vi "Versa_06.vi"() -> ()   [LabVIEW 2020]
uses:
  Visualisierungs Elemente/Zahlen-Ausgabefeld.ctl
  Funktionstasten/Funktionstasten.ctl
  Visualisierungs Elemente/Button.ctl
  Visualisierungs Elemente/String - Ausgabefeld.ctl
  IAG-Logo-A2.ctl
  Funktionstasten/Samplepoint Auswahlfeld.ctl
  Status Analysatoren/Status Analysatoren_Anzeige.ctl
  Seiten/FT-IR/FGV FT-IR Aktionen.ctl
  Funktionstasten/Funktionstasten-Aktion.ctl
  Passwortverwaltung/FGV Passwort Aktion.ctl
  Status Analysatoren/Aktion Status Analysatoren.ctl
  Auto Kalibrieren/Aktionen Zeitstempel speichern.ctl
  Seiten/Erweiterte Konfig/Aktion LN2 Extern Befuellung Warnung.ctl
  Seiten/System Einstellungen V2/Aktioen FGV System Konstanten.ctl
  SysLog/Aktionen FGV SysLog.ctl
  Funktionstasten/Zustaende.ctl
  Funktionstasten/Freigabe Aktionen.ctl
  Sprachverwaltung/FGV Aktion Tabelle zerlegen.ctl
  Allgemein/Aktion FGV Aufheizphase.ctl
  Allgemein/AufheizphaseCluster.ctl
  SysLog/SysLog Interface.ctl
  Funktionstasten/Aktionen Zustaende Loggen.ctl
  Stoerungen/Stoerungen Messgeraet/Aktionen Kommunikation Stoerung.ctl
  Allgemein/Aktionen Daten am cRIO speichern.ctl
  Seiten/Erweiterte Konfig/Aktionen LN2 Dewar Spuelen.ctl
  EPA 1065/Allgemeine VIs/Aktion Test Status.ctl
  <vilib>/event_ctls.llb/eventvkey.ctl
  Seiten/Log Konfig/Aktionen Trigger.ctl
  Bildwechsel/Bild-Auswahl.ctl
  Seiten/Anlagengrenzwerte/Aktion Durchflussaenderung.ctl
  Seiten/EL3000/FID/Aktion STY_MES.ctl
  Funktionstasten/FGV Erweiterte Bedienung Aktion.ctl
  AK-Schnittstelle/AK SATK Aktion.ctl
  Seiten/System Einstellungen V2/Aktioen FGV System.ctl
  Allgemein/Zykluszeiterfassung Aktionen.ctl
  Stoerungen/FGV Stoerungsdatei Aktionen.ctl
  Allgemein/Betriebsdaten Aktionen.ctl
  AK-Schnittstelle/AK Namen Aktionen.ctl
  Seiten/FT-IR/FGV FT-IR Gasliste Aktionen.ctl
  Seiten/CalGas Aufschaltung/FGV CalGas Aktionen.ctl
  Seiten/CalGas Aufschaltung/Cluster Auswahl Analysator.ctl
  Seiten/CalGas Aufschaltung/Analysator Auswahl.ctl
  Seiten/FT-IR/TOOLweb Interface Library/Trigger Aktionen.ctl
  Seiten/CalGas Aufschaltung/Definition CalGas Anzeige.ctl
  Seiten/CalGas Aufschaltung/CalGas-Namen.ctl
  Visualisierungs Elemente/String - Eingabefeld.ctl
  Seiten/CalGas Aufschaltung/CalGas-Werte.ctl
  Visualisierungs Elemente/Zahlen-Eingabefeld.ctl
  Seiten/CalGas Aufschaltung/CalGas-Einheit.ctl
  Visualisierungs Elemente/Auswahlfeld.ctl
  Seiten/CalGas Aufschaltung/CalGas-Messbereiche.ctl
  Schedule Modul/Aktion FGV Scheduler Status.ctl
  Stoerungen/FGV Stoermeldungen Aktion.ctl
  Allgemein/Bitte Warten.vi
  Passwortverwaltung/VI Passwortverwaltung.vi
  SysLog/SysLog Status.vi
  Sprachverwaltung/SprachEditor.vi
  Backup mit WebDAV/Backup.vi
  Allgemein/SPRACHE.vi
  EPA 1065/Dichtheitstest 1065-345/Konfig Leak Check.vi
  EPA 1065/Interference verificaton 1065-366/VI Interference Konfig.vi
  EPA 1065/T90 1065-308/T90 Test Konfig.vi
  EPA 1065/Interference verificaton 1065-375/VI Interference Konfig.vi
  EPA 1065/Gas Analyzer Drift 1065-550/Drift Verification Konfig.vi
  Linearisierung V2/VI Linearisierung v2.vi
  EPA 1065/HovaCAL Interference verification/VI Interference Konfig.vi
  Allgemein/allgemeine Sub-VIs.lvlib
  Seiten/FT-IR/TOOLweb Interface Library/TOOLweb Interface.lvlib
  Passwortverwaltung/Passwort.lvlib
  Funktionstasten/Funktionstasten.lvlib
  Bildwechsel/Bildwechsel.lvlib
  cRIO/PC/Kommunikation mit cRIO.lvlib
  Seiten/FT-IR/FT-IR.lvlib
  Seiten/FT-IR/TOOLweb Interface Library/Typdefinitionen.lvlib
  Seiten/Gaszuordnung AO/Gaszuordnung AO.lvlib
  Stoerungen/Stoerungen.lvlib
  Messdaten/Messdaten.lvlib
  AK-Schnittstelle/AK-Schnittstelle.lvlib
  Seiten/Log Konfig/LogKonfig.lvlib
  PNS/Komm Modbus/Komm Modbus.lvlib
  Seiten/Erweiterte Konfig/Erweiterte Konfig.lvlib
  cRIO Ueberwachung/cRIO Ueberwachung.lvlib
  Seiten/System Einstellungen V2/System Einstellungen V2.lvlib
  EPA 1065/Dichtheitstest 1065-345/Dichtheitstest 1065-345.lvlib
  Sprachverwaltung/Sprachverwaltung.lvlib
  Status Analysatoren/Status Analysatoren.lvlib
  Seiten/EL3000/FID/FID.lvlib
  Seiten/EL3000/PMA/PMA.lvlib
  Amium PNS/AK Kommunikation/AK Kommunikation.lvlib
  SysLog/SysLog.lvlib
  Backup mit WebDAV/Backup.lvlib
  Amium PNS/Amium PNS.lvlib
  Amium PNS/Aktion FGV Amium Daten.ctl
  Auto Kalibrieren/VI Auto Kalibrieren.vi
  Auto Kalibrieren/Auto Kalibrieren.lvlib
  Linearisierung V2/Gasteiler/Gasteiler.lvlib
  Linearisierung V2/Gasteiler/HovaCal/HovaCal.lvlib
  FTP WebDAV/FTP WebDAV.lvlib
  Seiten/CalGas Aufschaltung/CalGas Aufschaltung.lvlib
  Seiten/Anlagengrenzwerte/Anlagengrenzwerte.lvlib
  EPA 1065/ANR Test 1065-305/ARN Test 1065-305.lvlib
  EPA 1065/Interference verificaton 1065-366/Interference verificaton 1065-366.lvlib
  EPA 1065/T90 1065-308/T90 Test 1065-308.lvlib
  EPA 1065/EPA 1065.lvlib
  EPA 1065/Interference verificaton 1065-375/Interference verificaton 1065-375.lvlib
  Schedule Modul/Schedule Modul.lvlib
  EPA 1065/Gas Analyzer Drift 1065-550/Gas Analyzer Drift 1065-550.lvlib
  Linearisierung V2/Linearisierung v2.lvlib
  EPA 1065/HovaCAL Interference verification/HovaCAL Interference verificaton.lvlib
panel:
  out "Externe LN2 Warnung":string
  out "TestStatus":string
  in  "Aufschaltung Popup":bool
  in  "SystemLogListe":i32[](listbox)
  in  "SysLog":T1
  in  "Status Analysatoren":T2
  in  "LN2-Behälter Spülen":bool
  out "Letzte Kalibrierung":timestamp format="%<%H:%M:%S\n%x>T"
  out "LifeBit":bool
  in  "Betriebsart":u16(ring) items=["Manuell", "Remote", "Bitparallel"]
  out "Aktuelles Rezept":T3
  out "Datum und Uhrzeit":T3
  in  "login":T1
  out "PW-Level":T4 caption="Password-Level" format="%#_5g"
  in  "Funktionstasten":T5
  in  "Samplepoint":T6 items=["SP1"=1, "SP2"=2]
  in  "IAG":T7
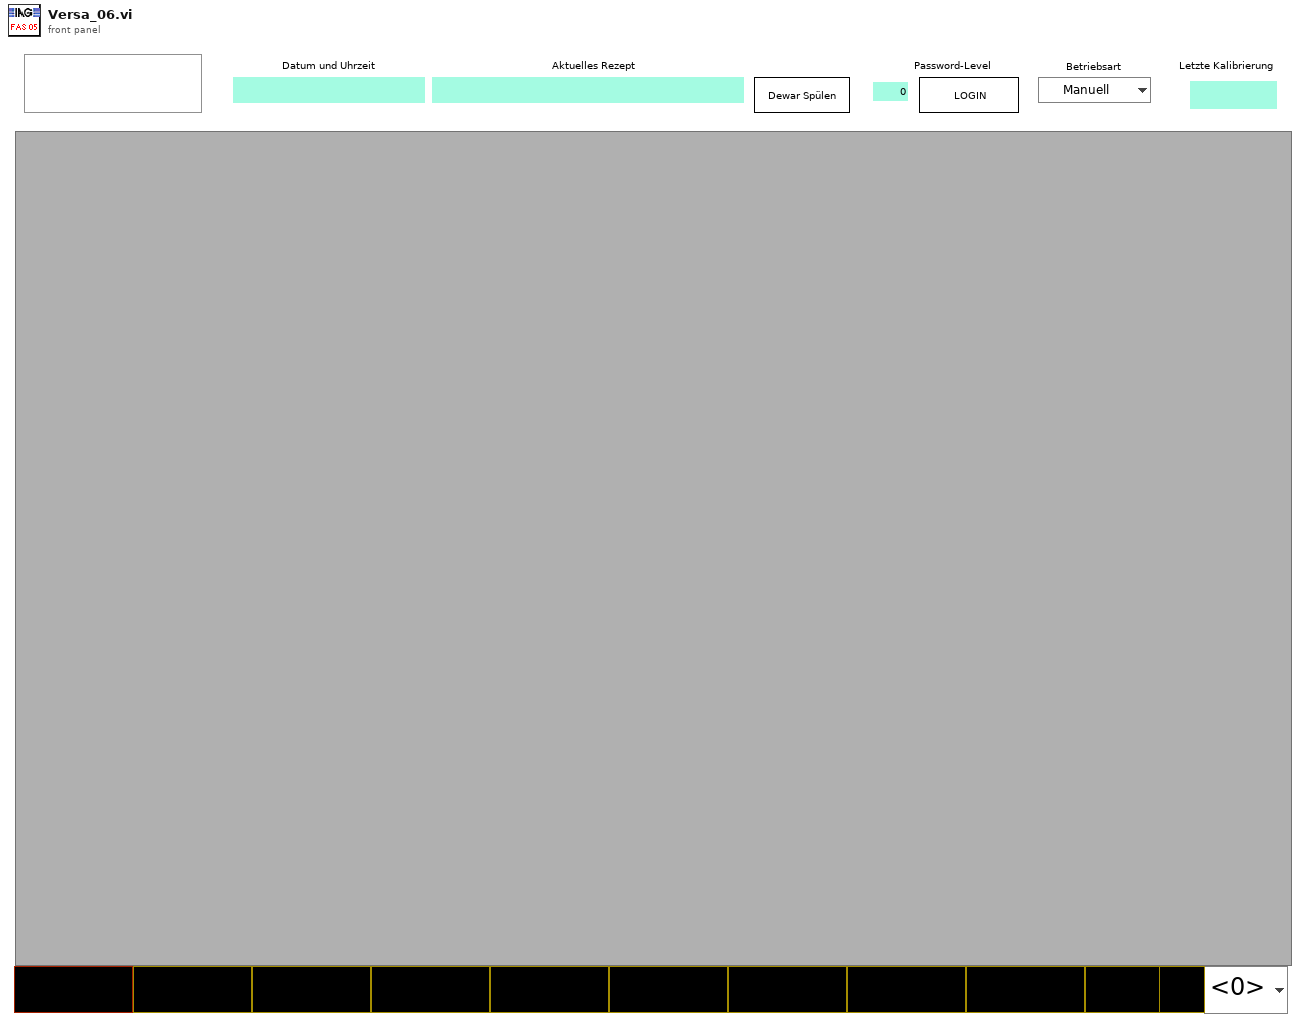
[diagram p1: front panel]
types:
  T1 = typedef "Button.ctl" = bool
  T2 = typedef "Status Analysatoren.lvlib/Status Analysatoren_Anzeige.ctl" = cluster{"FT-IR":bool, "FID":bool, "PMA":bool}
  T3 = typedef "String - Ausgabefeld.ctl" = string
  T4 = typedef "Zahlen-Ausgabefeld.ctl" = sgl
  T5 = typedef "Funktionstasten.lvlib/Funktionstasten.ctl" = cluster{"Taste 1":bool, "Taste 2":bool, "Taste 3":bool, "Taste 4":bool, "Taste 5":bool, "Taste 6":bool, "Taste 7":bool, "Taste 11":bool, "Taste 9":bool, "Taste 10":bool}
  T6 = typedef "Funktionstasten.lvlib/Samplepoint Auswahlfeld.ctl" = u16
  T7 = typedef "IAG-Logo-A2.ctl" = bool
  T8 = typedef "SysLog.lvlib/Aktionen FGV SysLog.ctl" = enum16{"initialisieren", "lesen", "schreiben", "history button ref", "Syslog_Anforderung"}
  T9 = typedef "Erweiterte Konfig.lvlib/Aktion LN2 Extern Befuellung Warnung.ctl" = enum16{"init", "blinken", "Warnungen ausgeben"}
  T10 = typedef "allgemeine Sub-VIs.lvlib/AufheizphaseCluster.ctl" = cluster{"FTIR":bool, "PNS Filterblock":bool, "Versa HL1":bool, "Versa HL2":bool, "PNS HL1":bool, "PNS HL2":bool, "PNS HL3":bool, "PNS HL4":bool, "HL zu FTIR":bool}
  T11 = typedef "allgemeine Sub-VIs.lvlib/Aktion FGV Aufheizphase.ctl" = enum16{"init", "lesen", "PNS Filterblock", "PNS HL1", "PNS HL2", "PNS HL3", "PNS HL4", "FTIR Messzelle", "HL 1", "HL 2", "HL zu FTIR", "auswerten"}
  T12 = typedef "Sprachverwaltung.lvlib/FGV Aktion Tabelle zerlegen.ctl" = enum16{"laden", "vereinzeln", "speichern"}
  T13 = typedef "Status Analysatoren.lvlib/Aktion Status Analysatoren.ctl" = enum16{"lesen", "initialisieren", "Analysatoren aktiv", "FTIR Fehler", "FID Fehler", "PMA Fehler", "Felder einfärben"}
  T14 = typedef "System Einstellungen V2.lvlib/Aktioen FGV System Konstanten.ctl" = enum16{"lesen", "laden", "speichern", "Sprache"}
  T15 = typedef "Funktionstasten.lvlib/Freigabe Aktionen.ctl" = enum16{"prüfen", "Freigabe?", "lesen"}
  T16 = typedef "Funktionstasten.lvlib/Zustaende.ctl" = enum16{"Standby", "Pause", "Eco", "Messen", "Kalibrieren", "Spülen Filter", "Spülen Leitung", "Umgebungsluft", "0-Gas", "Cal-Gas", "CG zu PNS", "-------------", "Init 1", "Init 2", "Init 3", "Init 4", "Messen vorbereiten", "Messen durchführen", "Exit"}
  T17 = typedef "Funktionstasten.lvlib/Funktionstasten-Aktion.ctl" = enum16{"Initialisieren", "Zustand setzen", "Taste gedrückt", "Fehler speichern", "Lesen", "Manuell", "Remote", "Bitparallel", "Samplepoint", "Zeit Prüfen", "reset Umschalten"}
  T18 = typedef "Funktionstasten.lvlib/Aktionen Zustaende Loggen.ctl" = enum16{"lesen", "schreiben", "löschen", "init"}
  T19 = typedef "SysLog.lvlib/SysLog Interface.ctl" = cluster{"FehlermeldungsCode":i32, "ErfolgsmeldungsCode":i32, "ParameterListenString":string, "Anzeige":bool, "SysLogIcon":enum16{"OK", "Warnung", "Fehler"}, "intern":bool}
  T20 = cluster{"Modell":string, "ProjektNummer":string, "Software Version":string, "Seriennummer":string}
  T21 = typedef "allgemeine Sub-VIs.lvlib/Aktionen Daten am cRIO speichern.ctl" = enum16{"lesen", "speichern setzen", "speichern reset", "gespeichert"}
  T22 = cluster{"Anzeige Array":bool[], "Message Array":string[], "SysLog Incon Array":enum16{"OK", "Warnung", "Fehler"}[], "Status Message Array":string[], "Status SysLog Incon Array":enum16{"OK", "Warnung", "Fehler"}[]}
  T23 = typedef "EPA 1065.lvlib/Aktion Test Status.ctl" = enum16{"init", "lesen", "prüfen", "Interference 366", "Interference 375", "Chiller läuft", "Drift läuft", "Pre Test läuft", "FID Optimization läuft", "FID Interference läuft", "HovaCAL Interference", "LinV2"}
  T24 = typedef "Erweiterte Konfig.lvlib/Aktionen LN2 Dewar Spuelen.ctl" = enum16{"lesen", "schreiben", "prüfen"}
  T25 = typedef "System Einstellungen V2.lvlib/Aktioen FGV System.ctl" = enum16{"lesen", "laden", "speichern", "Optionen schreiben", "Zeitstempel", "Reset BMP", "Reset SQP", "Wartung", "Werkseinstellung"}
  T26 = typedef "Amium PNS.lvlib/Aktion FGV Amium Daten.ctl" = enum16{"lesen", "Komm Daten", "Daten", "Error", "Regler", "Grenzwerte", "laden", "speichern"}
  T27 = typedef "eventvkey.ctl" = enum16{"ASCII", "Enter", "Return", "Shift", "Ctrl", "Alt", "Cmd", "Opt", "Caps", "NumLock", "Clear", "Break", "Up", "Down", "Left", "Right", "Insert", "Delete", "Home", "End", "PageUp", "PageDown", "Escape", "Help", "Pause", "ScrollLock", "F1", "F2", "F3", "F4", "F5", "F6", "F7", "F8", "F9", "F10", "F11", "F12", "F13", "F14", "F15", "F16", "F17", "F18", "F19", "F20", "F21", "F22", "F23", "F24", "Play", "VolumeUp", "VolumeDown", "Mute", "Two Byte Char"}
  T28 = typedef "LogKonfig.lvlib/Aktionen Trigger.ctl" = enum16{"lesen", "ALLE schreiben", "Trigger prüfen", "Trigger rücksetzen"}
  T29 = typedef "Bildwechsel.lvlib/Bild-Auswahl.ctl" = enum16{"lesen", "Initialisieren", "Beenden", "Grafik", "Anlagenübersicht", "Anlagengrenzwerte", "Log Konfig", "Gaszuordnung AO", "Erw. Konfiguration", "FT-IR  ", "Störmeldungen", "Störmeldepuffer", "Störmeldekonfig", "PNS Grenzwerte", "Statusübersicht", "Linearisierung", "ARN", "EPA Dichtheitstest", "FID", "PMA", "CalGas", "Lambda", "Interference", "Amium PNS", "EPA T90", "Interference N2O", "Scheduler", "Systemeinstellungen", "EPA Drift", "CAN Konfig", "HovaCAL Interference"}
  T30 = typedef "Passwort.lvlib/FGV Passwort Aktion.ctl" = enum16{"prüfen", "setzen", "Initialisieren", "PW speichern", "lesen", "PW Änderung"}
  T31 = typedef "Anlagengrenzwerte.lvlib/Aktion Durchflussaenderung.ctl" = enum16{"lesen", "Statusänderung", "Reset"}
  T32 = typedef "Aktion STY_MES.ctl" = enum16{"lesen", "setze STY", "setze MES", "MODBUS schreiben"}
  T33 = typedef "AK-Schnittstelle.lvlib/AK SATK Aktion.ctl" = enum16{"initialisieren", "lesen", "schreiben"}
  T34 = typedef "Funktionstasten.lvlib/FGV Erweiterte Bedienung Aktion.ctl" = enum16{"Lesen", "Initialisieren", "N2 zu PNS", "Chart wechsel"}
  T35 = typedef "FT-IR.lvlib/FGV FT-IR Aktionen.ctl" = enum16{"lesen", "NOG setzen", "NOS setzen", "Initialisieren", "speichern", "ALLES setzen", "FT-IR Spektrum loggen", "Komm Stoppen", "Spektrum LogKonfig"}
  T36 = enum16{"startrun", "runonce", "stoprun", "pauserun", "resumerun", "takeback"}
  T37 = typedef "Stoerungen.lvlib/Aktionen Kommunikation Stoerung.ctl" = enum16{"lesen", "init", "FT-IR Komm", "FT-IR Betriebsart", "FT-IR Hintergrund", "cRIO Komm", "PNS Komm", "Dichtheitstest", "Life Bit", "FTIR Komm AK", "PMA Komm", "FID Komm", "PMA Cal", "FID Ch4 Cal", "FID THC Cal", "Cal Timeout", "VFS 1 Komm", "VFS 2 Komm", "VFS 3 Komm", "VFS 4 Komm", "TRE 08 Komm", "CG-Test vorzeitig", "CG-Test Span 1", "CG-Test Span 2", "CG-Test Span 3", "CG-Test Messgas", "CG-Test löschen", "Test", "Amium AK", "AK Recept konfig", "AK Name konfig", "AK EKFG konfig"}
  T38 = enum16{"Init", "scroll H aktiv", "scroll H inaktiv", "scroll V aktiv", "scroll V inaktiv"}
  T39 = typedef "allgemeine Sub-VIs.lvlib/Zykluszeiterfassung Aktionen.ctl" = enum16{"lesen", "init", "Messdaten1", "ToolWeb", "AK FT-IR", "AK Extern", "AK Amium"}
  T40 = typedef "Stoerungen.lvlib/FGV Stoerungsdatei Aktionen.ctl" = enum16{"lesen", "laden", "Neue Werte"}
  T41 = typedef "allgemeine Sub-VIs.lvlib/Betriebsdaten Aktionen.ctl" = enum16{"Laden", "Speichern"}
  T42 = typedef "FT-IR.lvlib/FGV FT-IR Gasliste Aktionen.ctl" = enum16{"lesen", "Gasliste FT-IR", "Gasliste ausgelesen", "laden", "speichern", "löschen"}
  T43 = typedef "AK-Schnittstelle.lvlib/AK Namen Aktionen.ctl" = enum16{"lesen", "laden", "speichern Namen", "AK Namen", "Liste erstellen", "EKFG erstellen", "speichern EKFG", "EKFG schreiben", "Neuen Eintrag erzeugen"}
  T44 = typedef "CalGas Aufschaltung.lvlib/FGV CalGas Aktionen.ctl" = enum16{"lesen", "Analysator Auswahl", "Def.CalGas", "Aufschaltung CalGas", "laden", "speichern", "KAL extrahieren"}
  T45 = typedef "CalGas Aufschaltung.lvlib/Cluster Auswahl Analysator.ctl" = cluster{"Analysator Auswahl":T46, "Analysator Auswahl 2":T46, "Analysator Auswahl 3":T46, "Analysator Auswahl 4":T46, "Analysator Auswahl 5":T46, "Analysator Auswahl 6":T46, "Analysator Auswahl 7":T46, "Analysator Auswahl 8":T46, "Analysator Auswahl 9":T46, "Analysator Auswahl 10":T46, "Analysator Auswahl 11":T46, "Analysator Auswahl 12":T46}
  T46 = typedef "CalGas Aufschaltung.lvlib/Analysator Auswahl.ctl" = u16
  T47 = typedef "Schedule Modul.lvlib/Aktion FGV Scheduler Status.ctl" = enum16{"lesen", "init", "aktiv", "inaktiv"}
  T48 = typedef "CalGas Aufschaltung.lvlib/Definition CalGas Anzeige.ctl" = cluster{"Namen":T49, "Werte":T51, "Werte 2":T51, "Einheit":T53, "Messbereiche":T55}
  T49 = typedef "CalGas Aufschaltung.lvlib/CalGas-Namen.ctl" = cluster{"Name":T50, "Name 2":T50, "Name 3":T50, "Name 4":T50, "Name 5":T50, "Name 6":T50, "Name 7":T50, "Name 8":T50, "Name 9":T50, "Name 10":T50, "Name 11":T50, "Name 12":T50}
  T50 = typedef "String - Eingabefeld.ctl" = string
  T51 = typedef "CalGas Aufschaltung.lvlib/CalGas-Werte.ctl" = cluster{"Konzentration 1":T52, "Konzentration 2":T52, "Konzentration 3":T52, "Konzentration 4":T52, "Konzentration 5":T52, "Konzentration 6":T52, "Konzentration 7":T52, "Konzentration 8":T52, "Konzentration 9":T52, "Konzentration 10":T52, "Konzentration 11":T52, "Konzentration 12":T52}
  T52 = typedef "Zahlen-Eingabefeld.ctl" = sgl
  T53 = typedef "CalGas Aufschaltung.lvlib/CalGas-Einheit.ctl" = cluster{"Einheit 1":T54, "Einheit 2":T54, "Einheit 3":T54, "Einheit 4":T54, "Einheit 5":T54, "Einheit 6":T54, "Einheit 7":T54, "Einheit 8":T54, "Einheit 9":T54, "Einheit 10":T54, "Einheit 11":T54, "Einheit 12":T54}
  T54 = typedef "Auswahlfeld.ctl" = u16
  T55 = typedef "CalGas Aufschaltung.lvlib/CalGas-Messbereiche.ctl" = cluster{"Messbereich 1":T54, "Messbereich 2":T54, "Messbereich 3":T54, "Messbereich 4":T54, "Messbereich 5":T54, "Messbereich 6":T54, "Messbereich 7":T54, "Messbereich 8":T54, "Messbereich 9":T54, "Messbereich 10":T54, "Messbereich 11":T54, "Messbereich 12":T54}
  T56 = typedef "FT-IR.lvlib/TOOLweb Interface.lvlib/Typdefinitionen.lvlib/Trigger Aktionen.ctl" = enum16{"startrun", "runonce", "stoprun", "pauserun", "resumerun", "takeback"}
  T57 = typedef "Stoerungen.lvlib/FGV Stoermeldungen Aktion.ctl" = enum16{"Initialisieren", "kommend", "gehend", "lesen", "Queue leeren", "Queue freigeben", "in Datei loggen", "Änderung zurücksetzen"}
  T58 = typedef "Funktionstasten.lvlib/Betriebsart.ctl" = enum16{"Manuell", "Remote", "Bitparallel"}
  T59 = typedef "Amium PNS.lvlib/Daten Cluster.ctl" = cluster{"Amium Zustände":T60, "Samplepoint am PNS":i16, "Gerätekennung":string, "aktiver Samplepoint":i16[], "Messgasdruck":sgl}
  T60 = typedef "Amium PNS.lvlib/Amium Zustand.ctl" = u16
  T61 = typedef "System Einstellungen V2.lvlib/Optionen.ctl" = cluster{"Störmeldep.":bool, "Betriebszustände":bool, "AK in ppm":bool, "log Cal-Gas":bool, "log 0-Gas":bool, "Durchflusssensor 0-5V":bool, "PNS?":bool, "Mit N2 spülen":bool, "TRE08":bool, "Amium 10-Fach":bool, "Verticale Scrollbar aktiv":bool, "Loggingtakt":bool, "AK Rezeptwechsel gleich wie MKS":bool, "NG ECO":bool}
  T62 = typedef "Status Analysatoren.lvlib/Status.ctl" = cluster{"FT-IR aktiv":bool, "FT-IR Fehler":bool, "FID aktiv":bool, "FID Fehler":bool, "PMA aktiv":bool, "PMA Fehler":bool}
  T63 = cluster{"(80) labEnabled":bool, "(81) labPath":path, "(82) labBaseName":string, "(83) labIndex":string, "Spektrum loggen aktiv?":bool}
  T64 = typedef "Stoerungen.lvlib/Stoerungen Messgeraete.ctl" = cluster{"FT-IR Komm":bool, "FT-IR Betriebsart":bool, "FT-IR Hintergrundscan":bool, "Dichtheitstest":bool, "cRIO Komm":bool, "PNS Komm":bool, "Life Bit":bool, "FT-IR AK Komm":bool, "PMA Komm":bool, "FID Komm":bool, "PMA Cal":bool, "FID CH4 Cal":bool, "FID THC Cal":bool, "Cal Timeout":bool, "VFS 1 Komm":bool, "VFS 2 Komm":bool, "VFS 3 Komm":bool, "VFS 4 Komm":bool, "TRE 08 Komm":bool, "CG-Test":bool, "CG-Test 1":bool, "CG-Test 2":bool, "CG-Test 3":bool, "Messgas - Eingang":bool, "Amium AK Komm":bool, "AK Rezept nicht konfiguriert ":bool, "AK Name nicht konfiguriert":bool, "AK EKFG nicht konfiguriert":bool}
  T65 = cluster{"FT-IR aktiv":bool, "FID aktiv":bool, "PMA aktiv":bool}
  T66 = typedef "Auto Kalibrieren.lvlib/Aktionen Zeitstempel speichern.ctl" = enum16{"lesen", "Zeitstempel NEU", "laden", "speichern"}
  T67 = enum8{"Enabled", "Disabled", "Disabled and Grayed Out"}
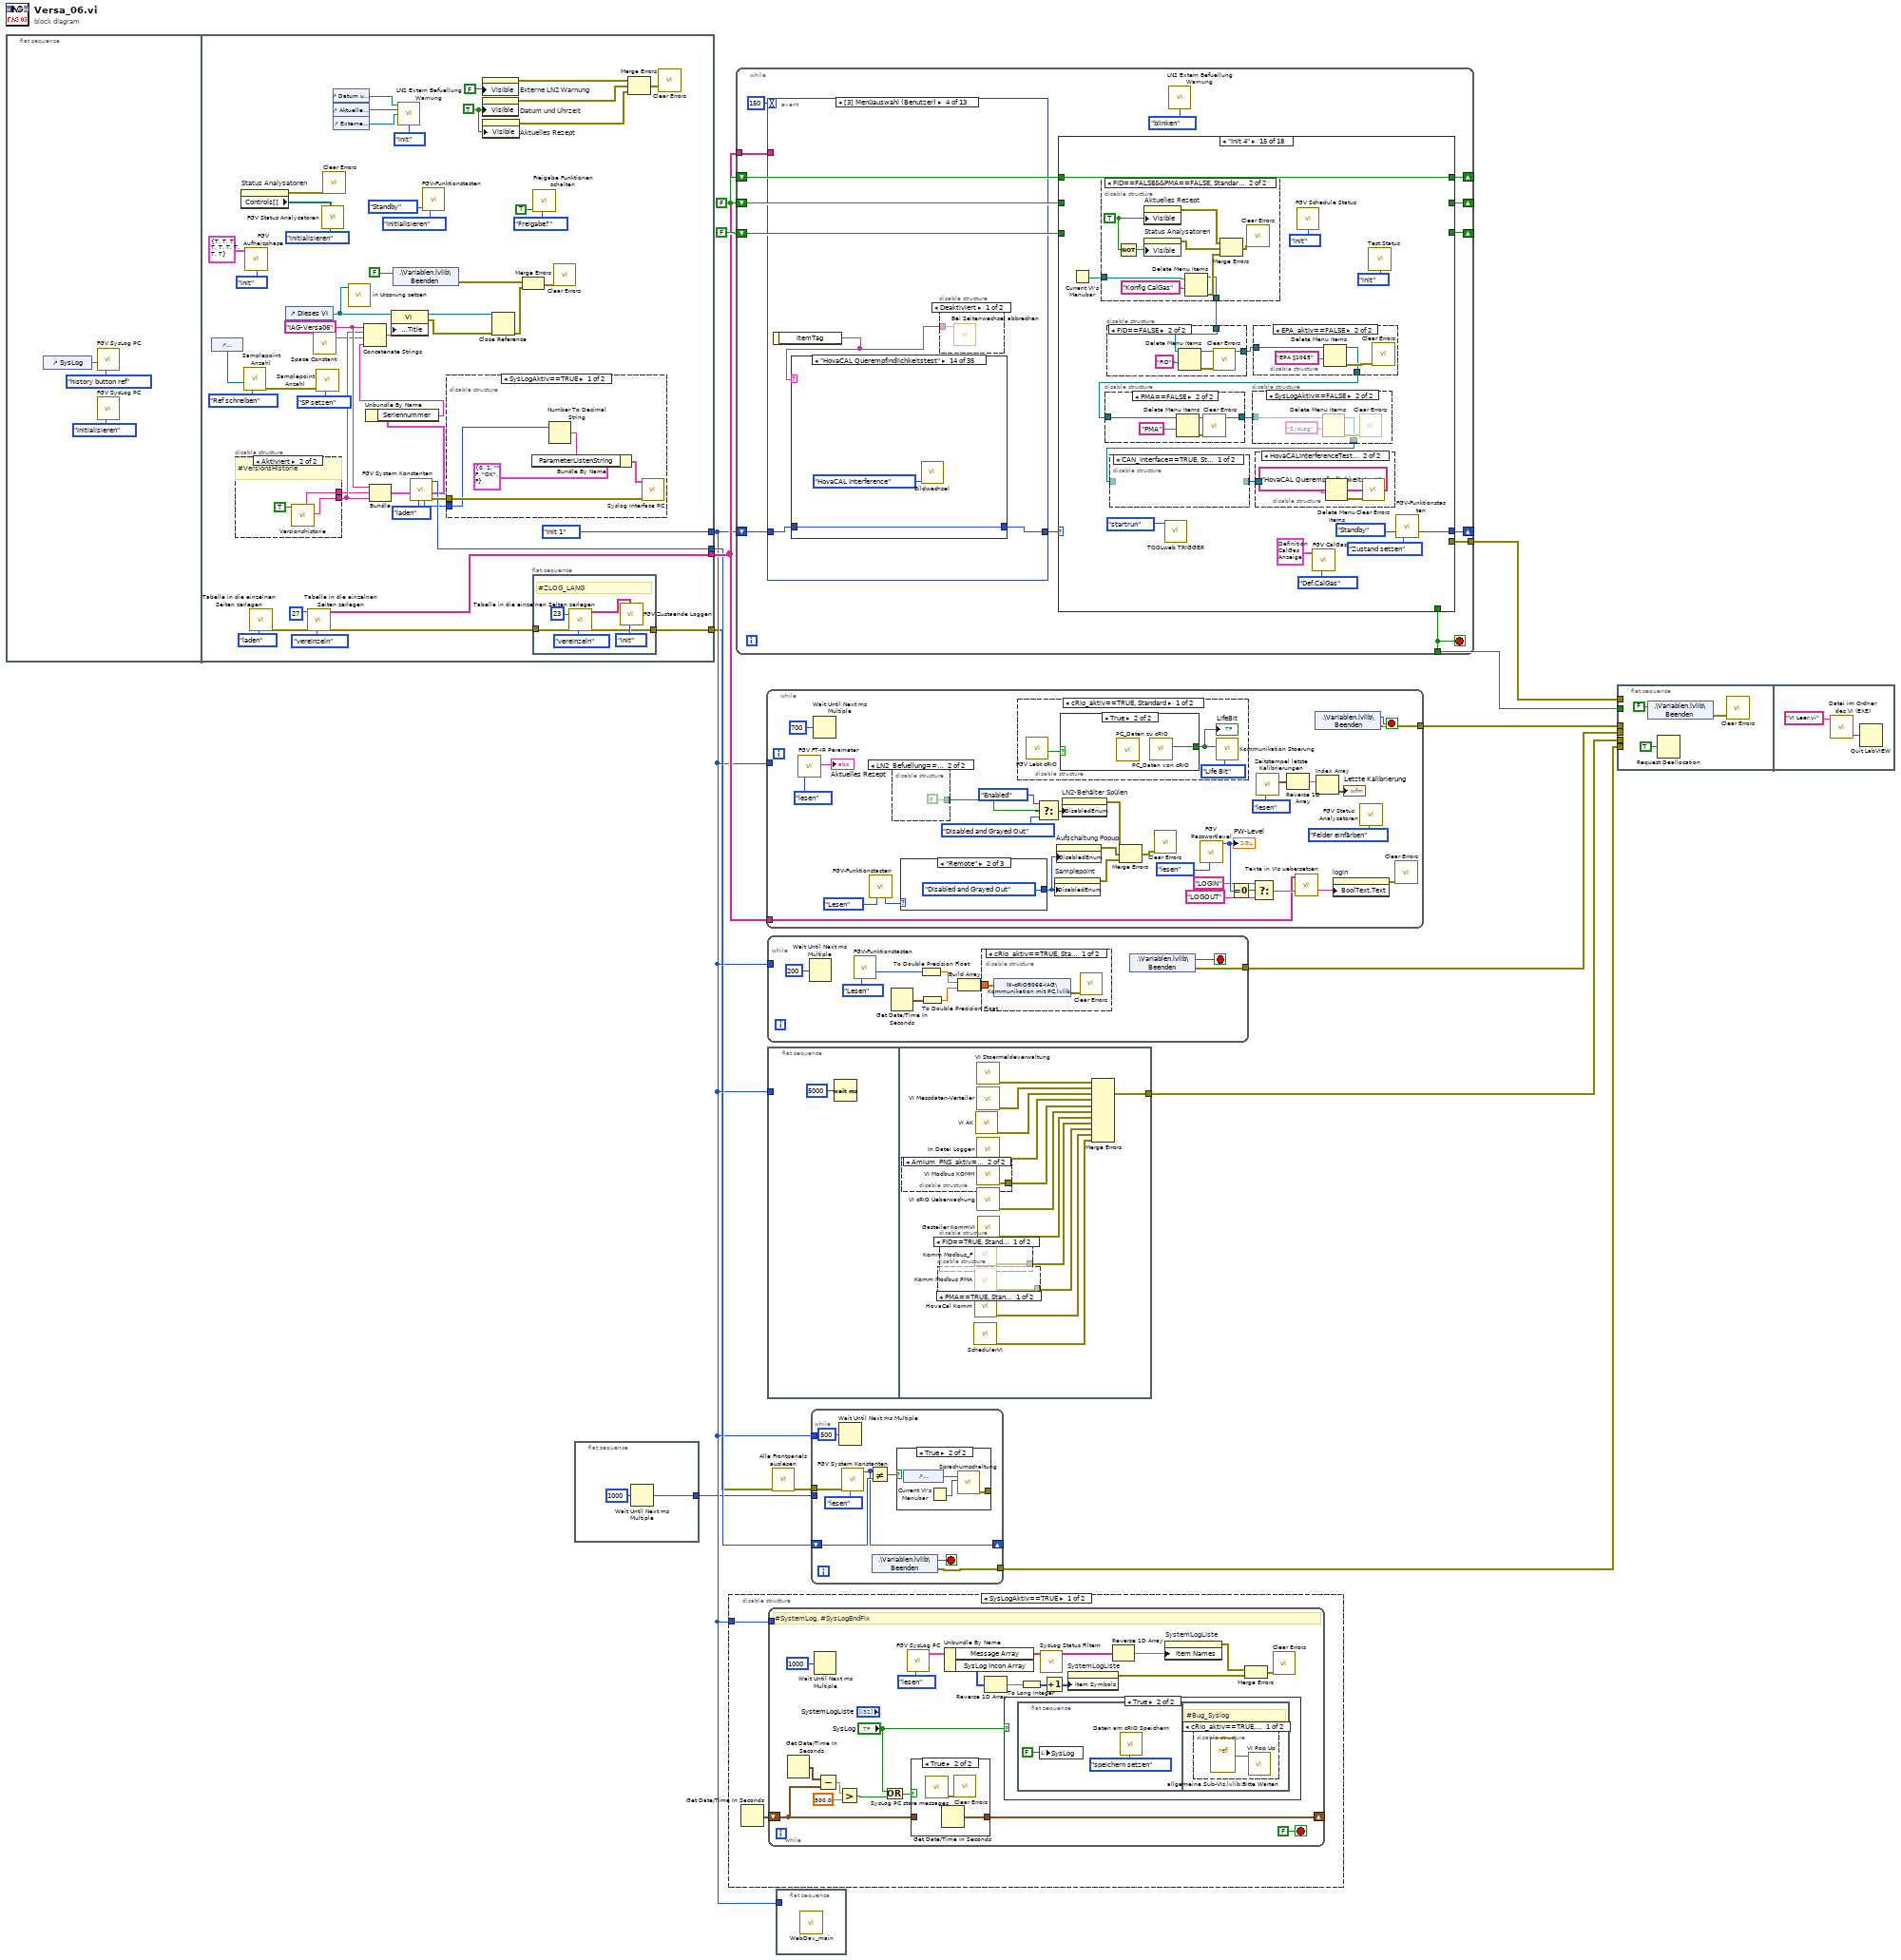
[diagram p0: block diagram]
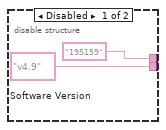
[diagram p7: hidden frame]
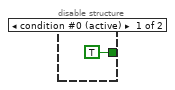
[diagram p10: hidden frame]
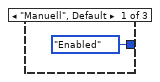
[diagram p13: hidden frame]
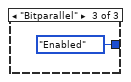
[diagram p14: hidden frame]
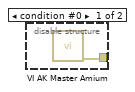
[diagram p17: hidden frame]
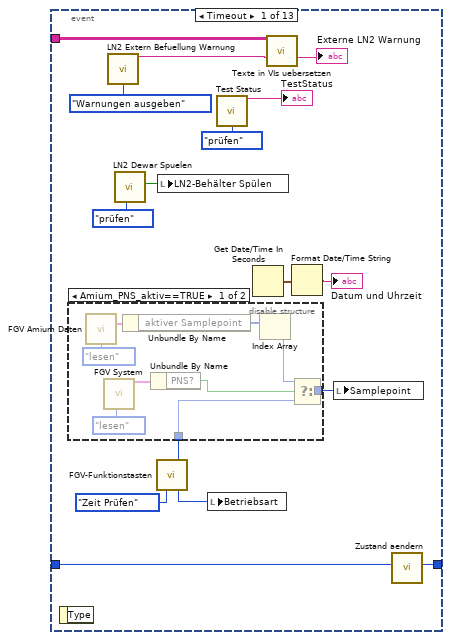
[diagram p18: hidden frame]
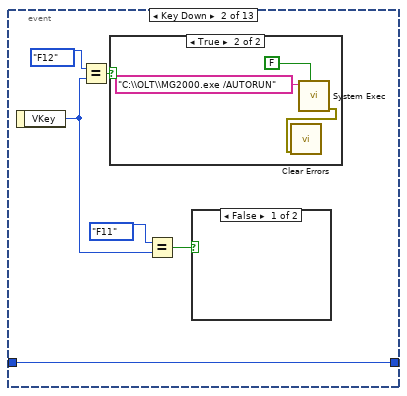
[diagram p20: hidden frame]
diagram:
  w9 = FALSE ("Freigabe?")
  n1 = flat-sequence {
    tunnel: [Zustaende."Init 1" ("Zustand")] -> w4
    tunnel: [w36] -> w7
    tunnel: [w41] -> w5
    tunnel: [w18] -> w1
    frame #0 {
      n2 = control-ref of="SysLog"() -> (w15:refnum<vi>)
      n3 = call "FGV SysLog PC.vi"("Aktion"=Aktionen_FGV_SysLog."history button ref", "Main History Button Referenz in"=w15) -> ()  [unwired: 5 in, 5 out]
      n4 = call "FGV SysLog PC.vi"("Aktion"=Aktionen_FGV_SysLog."initialisieren") -> ()  [unwired: 6 in, 5 out]
    }
    frame #1 {
      w24 = TRUE ("Sichtbar")
      w46 = "IAG-Versa06"
      n5 = control-ref of="Samplepoint"() -> (w38:refnum<vi>)
      n6 = disable-structure shown="Aktiviert" {
        disable-tunnel: [w75 w77] -> w45
        disable-tunnel: ["195159" w78] -> w44
        frame Disabled {
          w75 = "v4.9"  # Software Version
        }
        frame Enabled {
          # "#VersionsHistorie"
          n7 = call "Versionshistorie.vi"("Abfrage"=TRUE ("Hinweis aus")) -> ("v-PC"=w77:string, "Projekt"=w78:string)  [unwired: 8 in, 1 out]
        }
      }
      n8 = property on="Status Analysatoren" class="Cluster (strikt)"() -> (error out=w53:errorcluster, "Controls[]"=w51:refnum<vi>[])  [unwired: 2 in, 1 out]
      n9 = call "Samplepoint Anzahl.vi"("Aktion"=enum16{"lesen", "Ref schreiben", "SP setzen"}."Ref schreiben", "Samplepoint Referenz"=w38) -> ("error out"=w32:errorcluster)  [unwired: 8 in, 1 out]
      n10 = call "FGV Aufheizphase.vi"("Status"=T10 {"FTIR"=TRUE, "PNS Filterblock"=TRUE, "Versa HL1"=TRUE, "Versa HL2"=TRUE, "PNS HL1"=TRUE, "PNS HL2"=TRUE, "PNS HL3"=TRUE, "PNS HL4"=TRUE, "HL zu FTIR"=TRUE}, "Aktion"=Aktion_FGV_Aufheizphase."init") -> ()  [unwired: 11 in, 3 out]
      n11 = call "Tabelle in die einzelnen Seiten zerlegen.vi"("Aktion"=FGV_Aktion_Tabelle_zerlegen."laden") -> ("error out"=w48:errorcluster)  [unwired: 8 in, 2 out]
      n12 = control-ref of="Dieses VI"() -> (w42:refnum<vi>)
      n13 = call "Tabelle in die einzelnen Seiten zerlegen.vi"("Aktion"=FGV_Aktion_Tabelle_zerlegen."vereinzeln", "error in (no error)"=w48, "Index (Seite)"=27) -> ("error out"=w37:errorcluster, "Sprachliste"=w36:string[][])  [unwired: 6 in, 1 out]
      n14 = call <vilib>:"Space Constant.vi"() -> ("String"=w31:string)
      n15 = call "Samplepoint Anzahl.vi"("Aktion"=enum16{"lesen", "Ref schreiben", "SP setzen"}."SP setzen", "error in (no error)"=w32) -> ()  [unwired: 8 in, 2 out]
      n16 = call "FGV Status Analysatoren.vi"("Aktionen"=Aktion_Status_Analysatoren."initialisieren", "Controls[]"=w51) -> ()  [unwired: 9 in, 1 out]
      n17 = call <vilib>:"Clear Errors.vi"("error in (no error)"=w53) -> ()  [unwired: 5 in, 2 out]
      n18 = control-ref of="Datum und Uhrzeit"() -> (w20:refnum<vi>)
      n19 = control-ref of="Aktuelles Rezept"() -> (w19:refnum<vi>)
      n20 = control-ref of="Externe LN2 Warnung"() -> (w21:refnum<vi>)
      n21 = call "in Ursprung setzen.vi"("VI Referenz"=w42) -> ()  [unwired: 10 in, 1 out]
      n22 = Bundle(w46, "Projekt"=w44, "v-PC"=w45) -> (w43:cluster{string, "Projekt":string, "v-PC":string})  [unwired: 1 in]
      n23 = shared-variable ".\\Variablen.lvlib\\Beenden"(FALSE ("Beenden")) -> (error out=w57:errorcluster)  [unwired: 1 in]
      n24 = call "LN2 Extern Befuellung Warnung.vi"("Date and Time"=w20, "Rezept"=w19, "LN2 Warnung"=w21, "Aktion"=Aktion_LN2_Extern_Befuellung_Warnung."init") -> ()  [unwired: 10 in, 2 out]
      n25 = call "FGV System Konstanten.vi"("Aktionen"=Aktioen_FGV_System_Konstanten."laden", "Cluster in"=w43) -> ("error out"=w47:errorcluster, "Cluster out"=w30:T20, "Sprachindex"=w41:u16, "SysLogLevel"=w40:u32)  [unwired: 5 in, 1 out]
      n26 = Unbundle By Name(w30) -> ("Seriennummer"=w29:string)
      n27 = Concatenate Strings(w46, w45, w31, w29) -> (w59:string)
      n28 = property class="VI"(reference=w42, "Front Panel.Title"=w59) -> (reference out=w61:refnum<vi>, error out=w60:errorcluster)  [unwired: 1 in]
      n29 = call "FGV-Funktionstasten.vi"("Zustand"=Zustaende."Standby", "Aktion"=Funktionstasten-Aktion."Initialisieren") -> ()  [unwired: 6 in, 8 out]
      n30 = disable-structure shown="SysLogAktiv==TRUE" {
        disable-tunnel: w47 -> [w83 _]
        disable-tunnel: w40 -> [w81 _]
        frame condition #0 (active) {
          n31 = Number To Decimal String(number=w81) -> (decimal integer string=w79:string)  [unwired: 1 in]
          n32 = Bundle By Name(cluster=T19 {"FehlermeldungsCode"=0, "ErfolgsmeldungsCode"=1, "ParameterListenString"="", "Anzeige"=FALSE, "SysLogIcon"=enum."OK", "intern"=FALSE} ("Cluster (in)"), "ParameterListenString"=w79) -> (w80:T19)
          n33 = call "Syslog Interface PC.vi"("Fehler (in)"=w83, "Cluster (in)"=w80) -> ()  [unwired: 9 in, 1 out]
        }
        frame condition #1 {
        }
      }
      n34 = property on="Externe LN2 Warnung" class="Str"("Visible"=FALSE ("Sichtbar")) -> (error out=w26:errorcluster)  [unwired: 2 in, 1 out]
      n35 = property on="Datum und Uhrzeit" class="Str (strikt)"("Visible"=w24) -> (error out=w27:errorcluster)  [unwired: 2 in, 1 out]
      n36 = property on="Aktuelles Rezept" class="Str (strikt)"("Visible"=w24) -> (error out=w28:errorcluster)  [unwired: 2 in, 1 out]
      n37 = Close Reference(reference=w61, error in (no error)=w60) -> (error out=w56:errorcluster)
      n38 = Merge Errors(w57, w56) -> (w55:errorcluster)
      n39 = flat-sequence {
        tunnel: w37 -> [w72]
        tunnel: [w68] -> w18
        frame #0 {
          # "#ZLOG_LANG"
          n40 = call "Tabelle in die einzelnen Seiten zerlegen.vi"("Aktion"=FGV_Aktion_Tabelle_zerlegen."vereinzeln", "error in (no error)"=w72, "Index (Seite)"=23) -> ("error out"=w68:errorcluster, "Sprachliste"=w70:string[][])  [unwired: 6 in, 1 out]
          n41 = call "FGV Zustaende Loggen.vi"("Aktionen Zustände Loggen"=Aktionen_Zustaende_Loggen."init", "Sprachliste"=w70) -> ()  [unwired: 8 in, 2 out]
        }
      }
      n42 = call "Freigabe Funktionen schalten.vi"("Aktionen"=Freigabe_Aktionen."Freigabe?", "Freigabe?"=TRUE) -> ()  [unwired: 7 in, 3 out]
      n43 = call <vilib>:"Clear Errors.vi"("error in (no error)"=w55) -> ()  [unwired: 5 in, 2 out]
      n44 = Merge Errors(w26, w27, w28) -> (w25:errorcluster)
      n45 = call <vilib>:"Clear Errors.vi"("error in (no error)"=w25) -> ()  [unwired: 5 in, 2 out]
    }
  }
  n46 = flat-sequence {
    tunnel: [w84] -> w2
    frame #0 {
      n47 = Wait Until Next ms Multiple(millisecond multiple=u32 1000 ("ms")) -> (millisecond timer value=w84:u32)
    }
  }
  n48 = disable-structure shown="SysLogAktiv==TRUE" {
    disable-tunnel: w4 -> [w86 _]
    frame condition #0 (active) {
      n49 = Get Date/Time In Seconds() -> (seconds since 1Jan1904=w87:timestamp)
      n50 = while {
        shift-right: [w105] -> _
        shift-left: w87 -> [w104]
        tunnel: w86 -> [_]
        stop <- FALSE stop-if-true
        # "#SystemLog, #SysLogEndFix"
        n51 = Get Date/Time In Seconds() -> (seconds since 1Jan1904=w106:timestamp)
        n52 = Wait Until Next ms Multiple(millisecond multiple=u32 1000 ("Zu wartende ms")) -> ()  [unwired: 1 out]
        n53 = Subtract(x=w106, y=w104) -> (x-y=w107:dbl)
        n54 = Greater?(x=w107, y=300.0 ("Zu wartende ms")) -> (0:w101:bool)
        n55 = Or(x="SysLog", y=w101) -> (x .or. y?=w102:T1)
        n56 = call "FGV SysLog PC.vi"("Aktion"=Aktionen_FGV_SysLog."lesen") -> ("Anzeige Cluster"=w99:T22)  [unwired: 6 in, 4 out]
        n57 = case shown="True" w102 {
          tunnel: w104 -> [w113 _]
          tunnel: [w113 w115] -> w105
          frame False {
          }
          frame True {
            n58 = call "SysLog PC store messages.vi"() -> ("Fehler (out)"=w114:errorcluster)  [unwired: 11 in]
            n59 = Get Date/Time In Seconds() -> (seconds since 1Jan1904=w115:timestamp)
            n60 = call <vilib>:"Clear Errors.vi"("error in (no error)"=w114) -> ()  [unwired: 5 in, 2 out]
          }
        }
        n61 = Unbundle By Name(w99) -> ("Message Array"=w90:string[], "SysLog Incon Array"=w96:enum16{"OK", "Warnung", "Fehler"}[])
        n62 = Reverse 1D Array(array=w96) -> (reversed array=w98:enum16{"OK", "Warnung", "Fehler"}[])
        n63 = case shown="True" "SysLog" {
          frame False {
          }
          frame True {
            n64 = flat-sequence {
              frame #0 {
                n65 = local write "SysLog"(T1 FALSE ("SysLog")) -> ()
                n66 = call "Daten am cRIO Speichern.vi"("Aktionen"=Aktionen_Daten_am_cRIO_speichern."speichern setzen") -> ()  [unwired: 9 in, 2 out]
              }
              frame #1 {
                # "#Bug_Syslog"
                n67 = disable-structure shown="cRio_aktiv==TRUE, Standard" {
                  frame condition #0 (active) {
                    n68 = vi-ref "allgemeine Sub-VIs.lvlib:Bitte Warten.vi"() -> (w112:refnum<vi>)
                    n69 = call "VI Pop Up.vi"("VI Referenz"=w112) -> ()  [unwired: 10 in, 1 out]
                  }
                  frame condition #1 {
                  }
                }
              }
            }
          }
        }
        n70 = To Long Integer(number=w98) -> (32bit integer=w97:i32[])
        n71 = call "SysLog Status Filtern.vi"("Message Array"=w90) -> ("Message Array"=w89:string[])  [unwired: 10 in]
        n72 = Increment(x=w97) -> (x+1=w95:i32[])
        n73 = property on="SystemLogListe" class="Listenfeld (strikt)"("Item Symbols"=w95) -> (error out=w92:errorcluster)  [unwired: 2 in, 1 out]
        n74 = Reverse 1D Array(array=w89) -> (reversed array=w88:string[])
        n75 = property on="SystemLogListe" class="Listenfeld (strikt)"("Item Names"=w88) -> (error out=w93:errorcluster)  [unwired: 2 in, 1 out]
        n76 = Merge Errors(w93, w92) -> (w94:errorcluster)
        n77 = call <vilib>:"Clear Errors.vi"("error in (no error)"=w94) -> ()  [unwired: 5 in, 2 out]
      }
    }
    frame condition #1 {
    }
  }
  n78 = while {
    shift-right: [w127] -> _
    shift-left: w4 -> [w126]
    tunnel: [w125] -> w11
    shift-right: [w123] -> _
    shift-left: FALSE ("Freigabe?") -> [w124]
    shift-right: [w121] -> _
    shift-left: w9 -> [w122]
    shift-right: [w119] -> _
    shift-left: w9 -> [w120]
    tunnel: [w118] -> w8
    tunnel: w7 -> [w117]
    stop <- w125 stop-if-true
    n79 = event shown="[3] Menüauswahl (Benutzer)" {
      selector: _ -> [_ _ _ _ _ _ _ _ _ _ _ _ _]
      dyn-events: _ -> [_ _ _ _ _ _ _ _ _ _ _ _ _]
      timeout: 150 -> [_ _ _ _ _ _ _ _ _ _ _ _ _]
      tunnel: w126 -> [w141 w161 w168 w172 w271 w277 w283 w300 w302 w306 w316 w321 w330]
      tunnel: [w140 w161 w167 w171 w271 w277 w283 w300 w302 w307 w314 w321 w330] -> w128
      tunnel: w117 -> [w133 _ _ _ _ _ _ _ _ _ _ _ _]
      event Timeout {
        n80 = event-data() -> ()  [unwired: 2 out]
        n81 = call "LN2 Extern Befuellung Warnung.vi"("Aktion"=Aktion_LN2_Extern_Befuellung_Warnung."Warnungen ausgeben") -> ("Externe LN2 Warnung"=w130:string)  [unwired: 13 in, 1 out]
        n82 = call "LN2 Dewar Spuelen.vi"("Aktionen"=Aktionen_LN2_Dewar_Spuelen."prüfen") -> ("LN2 Spülen?"=w138:bool)  [unwired: 10 in]
        n83 = call "FGV-Funktionstasten.vi"("Aktion"=Funktionstasten-Aktion."Zeit Prüfen") -> ("Samplepoint"=w137:u16, "Betriebsart"=w142:T58)  [unwired: 7 in, 6 out]
        n84 = disable-structure shown="Amium_PNS_aktiv==TRUE" {
          disable-tunnel: w137 -> [w150 w155]
          disable-tunnel: [w149 w155] -> w136
          frame condition #0 {
            n85 = call "FGV Amium Daten.vi"("Aktion"=Aktion_FGV_Amium_Daten."lesen") -> ("Amium Daten"=w153:T59)  [unwired: 9 in, 5 out]
            n86 = call "FGV System.vi"("Aktionen"=Aktioen_FGV_System."lesen") -> ("Optionen"=w148:T61)  [unwired: 12 in, 6 out]
            n87 = Unbundle By Name(w153) -> ("aktiver Samplepoint"=w152:i16[])
            n88 = Unbundle By Name(w148) -> ("PNS?"=w146:bool)
            n89 = Index Array(array=w152) -> (element=w151:i16)  [unwired: 1 in]
            n90 = Select(t=w151, s=w146, f=w150) -> (s? t:f=w149:u16)
          }
          frame condition #1 (active) {
          }
        }
        n91 = local write "LN2-Behälter Spülen"(w138) -> ()
        n92 = local write "Betriebsart"(w142) -> ()
        n93 = call "Test Status.vi"("Aktion"=Aktion_Test_Status."prüfen") -> ("String"=→"TestStatus":string)  [unwired: 11 in, 3 out]
        n94 = Get Date/Time In Seconds() -> (seconds since 1Jan1904=w143:timestamp)
        n95 = call "Texte in VIs uebersetzen.vi"("Sprachliste"=w133, "String zum Übersetzen"=w130) -> ("String zum Übersetzen"=→"Externe LN2 Warnung":string)  [unwired: 9 in, 4 out]
        n96 = Format Date/Time String(seconds (now)=w143) -> (date/time string=→"Datum und Uhrzeit":string)  [unwired: 2 out]
        n97 = local write "Samplepoint"(w136) -> ()
        n98 = call "Zustand aendern.vi"("Zustand"=w141) -> ("Zustand"=w140:T16)  [unwired: 10 in]
      }
      event Key Down {
        n99 = event-data() -> ("VKey"=w156:T27)  [unwired: 1 out]
        n100 = Equal?(x=eventvkey."F12" ("VTaste"), y=w156) -> (x = y?=w159:bool)
        n101 = case shown="True" w159 {
          frame False {
          }
          frame True {
            n102 = call <vilib>:"System Exec.vi"("wait until completion? (T)"=FALSE, "command line"="C:\\OLT\\MG2000.exe /AUTORUN") -> ("error out"=w164:errorcluster)  [unwired: 6 in, 3 out]
            n103 = call <vilib>:"Clear Errors.vi"("error in (no error)"=w164) -> ()  [unwired: 5 in, 2 out]
          }
        }
        n104 = Equal?(x=eventvkey."F11" ("VTaste"), y=w156) -> (x = y?=w158:bool)
        n105 = case shown="False" w158 {
          frame False {
          }
          frame True {
            n106 = call "FGV Trigger.vi"("Aktion"=Aktionen_Trigger."Trigger prüfen", "Trigger setzen"=TRUE) -> ()  [unwired: 6 in, 4 out]
          }
        }
      }
      event Panel Close? {
        # "Filterereignis"
        n107 = event-data() -> ()  [unwired: 2 out]
        n108 = call "Runtime beenden.vi"("Zustand"=w168) -> ("Zustand"=w167:T16)  [unwired: 10 in]
        n109 = event-data("Discard?"=TRUE ("Verwerfen?")) -> ()  [unwired: 1 in, 1 out]
      }
      event Menu Selection (User) {
        n110 = event-data() -> ("ItemTag"=w170:string)  [unwired: 1 out]
        n111 = case shown="\"HovaCAL Querempfindlichkeitstest\"" w170 {
          tunnel: w172 -> [w174 w177 w181 w183 w185 w190 w195 w197 w199 w201 w203 w205 w207 w209 w211 w213 w215 w218 w220 w225 w230 w233 w235 w237 w239 w241 w245 w248 w250 w252 w253 w258 w260 w263 w264]
          tunnel: [w174 w177 w181 w183 w185 w190 w195 w197 w199 w201 w203 w205 w207 w209 w211 w213 w215 w218 w220 w225 w230 w233 w235 w237 w239 w241 w245 w248 w249 w252 w253 w258 w260 w263 w264] -> w171
          frame "Grafik" {
            n112 = call "Bildwechsel.vi"("nächstes Bild"=Bild-Auswahl."Grafik") -> ()  [unwired: 3 in, 8 out]
          }
          frame "Anlagenübersicht" {
            n113 = call "Bildwechsel.vi"("nächstes Bild"=Bild-Auswahl."Anlagenübersicht") -> ()  [unwired: 3 in, 8 out]
          }
          frame "Anlagengrenzwerte" {
            n114 = call "FGV Passwortlevel.vi"("FGV Passwort Aktion"=FGV_Passwort_Aktion."prüfen", "geforderter Level"=i16 5) -> ("Freigabe"=w178:bool)  [unwired: 2 in, 7 out]
            n115 = case shown="True" w178 {
              frame False {
              }
              frame True {
                n116 = call "Bildwechsel.vi"("nächstes Bild"=Bild-Auswahl."Anlagengrenzwerte") -> ()  [unwired: 3 in, 8 out]
              }
            }
          }
          frame "Log Konfig" {
            n117 = call "Bildwechsel.vi"("nächstes Bild"=Bild-Auswahl."Log Konfig") -> ()  [unwired: 3 in, 8 out]
          }
          frame "Gaszuordnung AO" {
            n118 = call "Bildwechsel.vi"("nächstes Bild"=Bild-Auswahl."Gaszuordnung AO") -> ()  [unwired: 3 in, 8 out]
          }
          frame "Erw. Konfiguration", Default {
            n119 = call "FGV Passwortlevel.vi"("FGV Passwort Aktion"=FGV_Passwort_Aktion."prüfen", "geforderter Level"=i16 5) -> ("Freigabe"=w187:bool)  [unwired: 2 in, 7 out]
            n120 = case shown="True" w187 {
              frame False {
              }
              frame True {
                n121 = call "Bildwechsel.vi"("nächstes Bild"=Bild-Auswahl."Erw. Konfiguration") -> ()  [unwired: 3 in, 8 out]
              }
            }
          }
          frame "Linearisierung" {
            n122 = call "FGV Passwortlevel.vi"("FGV Passwort Aktion"=FGV_Passwort_Aktion."prüfen", "geforderter Level"=i16 8) -> ("Freigabe"=w192:bool)  [unwired: 2 in, 7 out]
            n123 = case shown="True" w192 {
              frame False {
              }
              frame True {
                n124 = call "Bildwechsel.vi"("nächstes Bild"=Bild-Auswahl."Linearisierung") -> ()  [unwired: 3 in, 8 out]
              }
            }
          }
          frame "FT-IR" {
            n125 = call "Bildwechsel.vi"("nächstes Bild"=Bild-Auswahl."FT-IR  ") -> ()  [unwired: 3 in, 8 out]
          }
          frame "FID" {
            n126 = call "Bildwechsel.vi"("nächstes Bild"=Bild-Auswahl."FID") -> ()  [unwired: 3 in, 8 out]
          }
          frame "PMA" {
            n127 = call "Bildwechsel.vi"("nächstes Bild"=Bild-Auswahl."PMA") -> ()  [unwired: 3 in, 8 out]
          }
          frame "Konfig CalGas" {
            n128 = call "Bildwechsel.vi"("nächstes Bild"=Bild-Auswahl."CalGas") -> ()  [unwired: 3 in, 8 out]
          }
          frame "Lambda" {
            n129 = call "Bildwechsel.vi"("nächstes Bild"=Bild-Auswahl."Lambda") -> ()  [unwired: 3 in, 8 out]
          }
          frame "Querempfindlichkeitsnachweis §1065-366" {
            n130 = call "Bildwechsel.vi"("nächstes Bild"=Bild-Auswahl."Interference") -> ()  [unwired: 3 in, 8 out]
          }
          frame "HovaCAL Querempfindlichkeitstest" {
            n131 = call "Bildwechsel.vi"("nächstes Bild"=Bild-Auswahl."HovaCAL Interference") -> ()  [unwired: 3 in, 8 out]
          }
          frame "EPA Drift" {
            n132 = call "Bildwechsel.vi"("nächstes Bild"=Bild-Auswahl."EPA Drift") -> ()  [unwired: 3 in, 8 out]
          }
          frame "Querempfindlichkeitsnachweis §1065-375" {
            n133 = call "Bildwechsel.vi"("nächstes Bild"=Bild-Auswahl."Interference N2O") -> ()  [unwired: 3 in, 8 out]
          }
          frame "PNS Grenzwerte" {
            n134 = disable-structure shown="Amium_PNS_aktiv==TRUE, Standard" {
              frame condition #0 {
                n135 = call "Bildwechsel.vi"("nächstes Bild"=Bild-Auswahl."Amium PNS") -> ()  [unwired: 3 in, 8 out]
              }
              frame condition #1 (active) {
                n136 = call "Bildwechsel.vi"("nächstes Bild"=Bild-Auswahl."PNS Grenzwerte") -> ()  [unwired: 3 in, 8 out]
              }
            }
          }
          frame "Statusübersicht" {
            n137 = call "Bildwechsel.vi"("nächstes Bild"=Bild-Auswahl."Statusübersicht") -> ()  [unwired: 3 in, 8 out]
          }
          frame "CAN Konfig" {
            n138 = call "Bildwechsel.vi"("nächstes Bild"=Bild-Auswahl."CAN Konfig") -> ()  [unwired: 3 in, 8 out]
          }
          frame "Einstellungen" {
            # "#SystemEinstellungenV2"
            n139 = call "FGV Passwortlevel.vi"("FGV Passwort Aktion"=FGV_Passwort_Aktion."prüfen", "geforderter Level"=i16 5) -> ("Freigabe"=w222:bool)  [unwired: 7 in, 2 out]
            n140 = case shown="True" w222 {
              frame False {
              }
              frame True {
                n141 = call "Bildwechsel.vi"("nächstes Bild"=Bild-Auswahl."Systemeinstellungen") -> ()  [unwired: 6 in, 5 out]
              }
            }
          }
          frame "Diagnose Steuerung" {
            n142 = call "FGV Passwortlevel.vi"("FGV Passwort Aktion"=FGV_Passwort_Aktion."prüfen", "geforderter Level"=i16 5) -> ("Freigabe"=w227:bool)  [unwired: 7 in, 2 out]
            n143 = case shown="True" w227 {
              frame False {
              }
              frame True {
                n144 = vi-ref "VI Fehlerliste.vi"() -> (w231:refnum<vi>)
                n145 = call "VI Pop Up.vi"("VI Referenz"=w231) -> ()  [unwired: 10 in, 1 out]
              }
            }
          }
          frame "Störmeldungen" {
            n146 = call "Bildwechsel.vi"("nächstes Bild"=Bild-Auswahl."Störmeldungen") -> ()  [unwired: 6 in, 5 out]
          }
          frame "ARN Test" {
            n147 = call "Bildwechsel.vi"("nächstes Bild"=Bild-Auswahl."ARN") -> ()  [unwired: 6 in, 5 out]
          }
          frame "EPA T90" {
            n148 = call "Bildwechsel.vi"("nächstes Bild"=Bild-Auswahl."EPA T90") -> ()  [unwired: 6 in, 5 out]
          }
          frame "Dichtheitstest" {
            n149 = call "Bildwechsel.vi"("nächstes Bild"=Bild-Auswahl."EPA Dichtheitstest") -> ()  [unwired: 6 in, 5 out]
          }
          frame "Störmeldepuffer" {
            n150 = call "Bildwechsel.vi"("nächstes Bild"=Bild-Auswahl."Störmeldepuffer") -> ()  [unwired: 6 in, 5 out]
          }
          frame "Konfig Störmeldungen" {
            n151 = call "FGV Passwortlevel.vi"("FGV Passwort Aktion"=FGV_Passwort_Aktion."prüfen", "geforderter Level"=i16 8) -> ("Freigabe"=w242:bool)  [unwired: 2 in, 7 out]
            n152 = case shown="True" w242 {
              frame False {
              }
              frame True {
                n153 = call "Bildwechsel.vi"("nächstes Bild"=Bild-Auswahl."Störmeldekonfig") -> ()  [unwired: 3 in, 8 out]
              }
            }
          }
          frame "Passwort Verwaltung" {
            n154 = vi-ref "Passwort.lvlib:VI Passwortverwaltung.vi"() -> (w247:refnum<vi>)
            n155 = call "VI Pop Up.vi"("VI Referenz"=w247) -> ()  [unwired: 10 in, 1 out]
          }
          frame "Beenden" {
            n156 = call "Runtime beenden.vi"("Zustand"=w250) -> ("Zustand"=w249:T16)  [unwired: 10 in]
          }
          frame "über" {
            n157 = vi-ref "VI Copyright.vi"() -> (w251:refnum<vi>)
            n158 = call "VI Pop Up.vi"("VI Referenz"=w251) -> ()  [unwired: 10 in, 1 out]
          }
          frame "SysLog" {
            n159 = vi-ref "SysLog.lvlib:SysLog Status.vi"() -> (w254:refnum<vi>)
            n160 = call "VI Pop Up.vi"("VI Referenz"=w254) -> ()  [unwired: 10 in, 1 out]
          }
          frame "Spracheditor" {
            n161 = call "FGV Passwortlevel.vi"("FGV Passwort Aktion"=FGV_Passwort_Aktion."prüfen", "geforderter Level"=i16 8) -> ("Freigabe"=w255:bool)  [unwired: 2 in, 7 out]
            n162 = case shown="True" w255 {
              frame False {
              }
              frame True {
                n163 = vi-ref "Sprachverwaltung.lvlib:SprachEditor.vi"() -> (w259:refnum<vi>)
                n164 = call "VI Pop Up.vi"("VI Referenz"=w259) -> ()  [unwired: 10 in, 1 out]
              }
            }
          }
          frame "Backup" {
            n165 = vi-ref "Backup.lvlib:Backup.vi"() -> (w261:refnum<vi>)
            n166 = call "VI Pop Up.vi"("VI Referenz"=w261) -> ()  [unwired: 10 in, 1 out]
          }
          frame "Scheduler" {
            n167 = call "Bildwechsel.vi"("nächstes Bild"=Bild-Auswahl."Scheduler") -> ()  [unwired: 3 in, 8 out]
          }
          frame "Linearity verification §1065-307" {
            n168 = call "FGV Passwortlevel.vi"("FGV Passwort Aktion"=FGV_Passwort_Aktion."prüfen", "geforderter Level"=i16 8) -> ("Freigabe"=w265:bool)  [unwired: 2 in, 7 out]
            n169 = case shown="True" w265 {
              frame False {
              }
              frame True {
                n170 = call "Bildwechsel.vi"("nächstes Bild"=Bild-Auswahl."Linearisierung") -> ()  [unwired: 3 in, 8 out]
              }
            }
          }
        }
        n171 = disable-structure shown="Deaktiviert" {
          disable-tunnel: w170 -> [w173 _]
          frame Disabled {
            n172 = call "Bei Seitenwechsel abbrechen.vi"("Menüstring"=w173) -> ()  [unwired: 11 in]
          }
          frame Enabled {
          }
        }
      }
      event "Aufschaltung Popup": Value Change {
        n173 = event-data() -> ()  [unwired: 2 out]
        n174 = vi-ref "CalGas Aufschaltung.lvlib:Aufschaltung_Popup.vi"() -> (w269:refnum<vi>)
        n175 = case shown="False" "Aufschaltung Popup" {
          tunnel: w269 -> [w272 w274]
          frame False {
            n176 = call "VI Shut Down.vi"("VI Referenz"=w272) -> ()  [unwired: 11 in]
          }
          frame True {
            n177 = call "VI Pop Up_Calgas-Popup.vi"("Zentrieren"=FALSE, "VI Referenz"=w274) -> ()  [unwired: 10 in]
          }
        }
      }
      event Panel Resize {
        n178 = event-data() -> ()  [unwired: 2 out]
        n179 = vi-ref "Aufschaltung_Popup.vi"() -> (w276:refnum<vi>)
        n180 = local write "Aufschaltung Popup"(FALSE ("Aufschaltung Popup")) -> ()
        n181 = call "VI Shut Down.vi"("VI Referenz"=w276) -> ()  [unwired: 11 in]
      }
      event Value Change {
        n182 = event-data() -> ("OldVal"=w278:T2, "NewVal"=w279:T2)  [unwired: 1 out]
        n183 = call "FGV Passwortlevel.vi"("FGV Passwort Aktion"=FGV_Passwort_Aktion."prüfen", "geforderter Level"=i16 5) -> ("Freigabe"=w280:bool)  [unwired: 2 in, 7 out]
        n184 = case shown="True" w280 {
          tunnel: w279 -> [_ w287]
          tunnel: w278 -> [w284 _]
          frame False {
            n185 = local write "Status Analysatoren"(w284) -> ()
          }
          frame True {
            n186 = stacked-sequence {
              tunnel: w287 -> [w295 _]
              frame #0 {
                n187 = Unbundle By Name(w295) -> ("FID"=w294:bool)
                n188 = Equal?(x=w294, y=FALSE) -> (x = y?=w290:bool)
                n189 = Not(x=w290) -> (.not. x?=w289:bool)
                n190 = call "STBY_MESSEN.vi"("Messen"=w289, "Aktion"=Aktion_STY_MES."setze MES") -> ()  [unwired: 10 in, 4 out]
                n191 = call "STBY_MESSEN.vi"("Standby"=w290, "Aktion"=Aktion_STY_MES."setze STY") -> ()  [unwired: 10 in, 4 out]
              }
              frame #1 {
                n192 = call "STBY_MESSEN.vi"("Case Nr."=2, "Aktion"=Aktion_STY_MES."MODBUS schreiben") -> ()  [unwired: 10 in, 4 out]
              }
            }
            n193 = call "FGV Status Analysatoren.vi"("Aktionen"=Aktion_Status_Analysatoren."Analysatoren aktiv", "Aktiv"=w287) -> ("Status Analysatoren"=w286:T62)  [unwired: 9 in]
            n194 = call "Durchfluss aendern bei Analysatorstatus.vi"("Aktion"=Aktion_Durchflussaenderung."Statusänderung", "Status Analysatoren"=w286) -> ()  [unwired: 8 in, 2 out]
          }
        }
      }
      event Value Change {
        n195 = event-data() -> ()  [unwired: 2 out]
        n196 = call "FGV-Funktionstasten.vi"("Samplepoint"="Samplepoint", "Aktion"=Funktionstasten-Aktion."Samplepoint") -> ()  [unwired: 6 in, 8 out]
      }
      event Value Change {
        # "#Sprachumschaltung"
        n197 = event-data() -> ()  [unwired: 2 out]
        n198 = disable-structure shown="Deaktiviert" {
          frame Disabled {
            n199 = call <vilib>:"System Exec.vi"("command line"="C:\\Programme\\HotVirtualKeyboard\\hvk.exe") -> ()  [unwired: 7 in, 4 out]
          }
          frame Enabled {
          }
        }
        n200 = disable-structure shown="Deaktiviert" {
          frame Disabled {
            n201 = call "Bildwechsel.vi"("nächstes Bild"=Bild-Auswahl."Störmeldungen") -> ()  [unwired: 3 in, 8 out]
          }
          frame Enabled {
          }
        }
        n202 = vi-ref "allgemeine Sub-VIs.lvlib:SPRACHE.vi"() -> (w301:refnum<vi>)
        n203 = call "VI Pop Up.vi"("VI Referenz"=w301) -> ()  [unwired: 10 in, 1 out]
      }
      event "Betriebsart": Value Change {
        n204 = event-data() -> ()  [unwired: 2 out]
        n205 = case shown="2" "Betriebsart" {
          tunnel: [w308 w310 w312] -> w307
          tunnel: w306 -> [w308 w310 w312]
          frame 0, Default {
            # "Manuell"
            n206 = call "FGV-Funktionstasten.vi"("Aktion"=Funktionstasten-Aktion."Manuell") -> ()  [unwired: 7 in, 8 out]
          }
          frame 1 {
            # "Remote"
            n207 = call "FGV-Funktionstasten.vi"("Aktion"=Funktionstasten-Aktion."Remote") -> ()  [unwired: 7 in, 8 out]
          }
          frame 2 {
            # "Bitparallel"
            n208 = call "FGV-Funktionstasten.vi"("Aktion"=Funktionstasten-Aktion."Bitparallel") -> ()  [unwired: 7 in, 8 out]
          }
        }
      }
      event Value Change {
        n209 = event-data() -> ()  [unwired: 2 out]
        n210 = call "FGV-Funktionstasten.vi"("Funktionstasten"="Funktionstasten", "Zustand"=w316, "Aktion"=Funktionstasten-Aktion."Taste gedrückt") -> ("ausgewählte Funktion"=w314:T16)  [unwired: 5 in, 7 out]
      }
      event Value Change {
        n211 = event-data() -> ()  [unwired: 2 out]
        n212 = local read "PW-Level"() -> (w319:T4)
        n213 = Increment(x=w319) -> (x+1=w318:T4)
        n214 = Equal To 0?(x=w319) -> (x = 0?=w320:bool)
        n215 = case shown="False" w320 {
          tunnel: w318 -> [w323 _]
          frame True {
            n216 = call "FGV Passwortlevel.vi"("FGV Passwort Aktion"=FGV_Passwort_Aktion."setzen", "geforderter Level"=w323) -> ("aktueller Level"=w324:i16)  [unwired: 2 in, 7 out]
            n217 = local write "PW-Level"(w324) -> ()
          }
          frame False {
            n218 = call "FGV Passwortlevel.vi"("FGV Passwort Aktion"=FGV_Passwort_Aktion."Initialisieren", "geforderter Level"=i16 0) -> ("aktueller Level"=w326:i16)  [unwired: 2 in, 7 out]
            n219 = local write "PW-Level"(w326) -> ()
          }
        }
      }
      event "LN2-Behälter Spülen": Value Change {
        n220 = event-data() -> ()  [unwired: 2 out]
        n221 = call "LN2 Dewar Spuelen.vi"("Aktionen"=Aktionen_LN2_Dewar_Spuelen."schreiben", "LN2 Spülen?"="LN2-Behälter Spülen") -> ()  [unwired: 9 in, 1 out]
        n222 = disable-structure shown="SysLogAktiv==TRUE" {
          disable-tunnel: "LN2-Behälter Spülen" -> [_ _]
          frame condition #0 (active) {
            n223 = call "Syslog Interface PC.vi"("Cluster (in)"=T19 {"FehlermeldungsCode"=2, "ErfolgsmeldungsCode"=2, "ParameterListenString"="", "Anzeige"=FALSE, "SysLogIcon"=enum."OK", "intern"=FALSE}) -> ()  [unwired: 10 in, 1 out]
          }
          frame condition #1 {
          }
        }
      }
    }
    n224 = case shown="\"Init 4\"" w128 {
      selector: w128 -> [w342 w354 w358 w370 _ w388 w390 w392 w397 w416 w432 _ _ _ _ w571 w577 w581]
      tunnel: [w342 w354 w358 w372 Zustaende."-------------" ("Zustand") w388 w390 w392 w397 w416 w432 Zustaende."Init 2" ("Zustand") Zustaende."Init 3" ("Zustand") Zustaende."Init 4" ("Zustand") w518 w570 w577 w581] -> w127
      tunnel: [_ _ _ _ _ _ _ _ _ _ _ _ _ _ _ _ _ w580] -> w125
      tunnel: w124 -> [_ _ _ _ _ _ _ _ w396 w415 _ _ _ _ _ _ _ _]
      tunnel: [_ _ _ _ _ _ _ _ w395 w414 _ _ _ _ _ _ _ _] -> w123
      tunnel: w122 -> [_ _ w357 _ _ _ _ _ _ _ _ _ _ _ _ _ _ _]
      tunnel: [_ _ w356 _ _ _ _ _ _ _ _ _ _ _ _ _ _ _] -> w121
      tunnel: w120 -> [w335 w353 _ w369 w376 w387 w389 w391 w393 w412 w431 w435 w441 w492 w516 w563 w576 w579]
      tunnel: [w334 w353 TRUE ("Freigabe?") w369 w376 w387 w389 w391 w393 w412 w431 w435 w441 w492 w516 w563 w576 w579] -> w119
      tunnel: [_ _ _ _ _ _ _ _ _ _ _ _ _ w468 _ _ _ w578] -> w118
      frame "Standby", Default {
        n225 = call "FGV FT-IR Parameter.vi"("Aktion"=FGV_FT-IR_Aktionen."lesen") -> ("Ausgangs-Cluster"=w338:T63)  [unwired: 11 in, 7 out]
        n226 = call "FGV Trigger.vi"("Aktion"=Aktionen_Trigger."Trigger rücksetzen") -> ()  [unwired: 7 in, 4 out]
        n227 = call "FGV-Erweiterte Bedienung.vi"("Aktion"=FGV_Erweiterte_Bedienung_Aktion."N2 zu PNS", "N2 zu PNS"=FALSE) -> ()  [unwired: 8 in, 2 out]
        n228 = Unbundle By Name(w338) -> ("(80) labEnabled"=w340:bool)
        n229 = case shown="True" w335 {
          selector: w335 -> [w343 _]
          tunnel: [w343 _] -> w334
          frame False {
          }
          frame True {
            # "Signal kommt von ECO"
            n230 = local read "Status Analysatoren"() -> (w345:T2)
            n231 = Unbundle By Name(w345) -> ("FID"=w344:bool)
            n232 = case shown="True" w344 {
              frame False {
              }
              frame True {
                n233 = stacked-sequence {
                  frame #0 {
                    w346 = FALSE ("Standby")
                    n234 = Not(x=w346) -> (.not. x?=w347:bool)
                    n235 = call "STBY_MESSEN.vi"("Messen"=w347, "Aktion"=Aktion_STY_MES."setze MES") -> ()  [unwired: 10 in, 4 out]
                    n236 = call "STBY_MESSEN.vi"("Standby"=w346, "Aktion"=Aktion_STY_MES."setze STY") -> ()  [unwired: 10 in, 4 out]
                  }
                  frame #1 {
                    n237 = call "STBY_MESSEN.vi"("Case Nr."=2, "Aktion"=Aktion_STY_MES."MODBUS schreiben") -> ()  [unwired: 10 in, 4 out]
                  }
                }
              }
            }
          }
        }
        n238 = case shown="True" w340 {
          frame False {
          }
          frame True {
            n239 = call "TOOLweb SET LABFILE Enabled.vi"("Enabled"=FALSE) -> ()  [unwired: 2 in, 5 out]
          }
        }
        n240 = call "AK SATK FGV.vi"("Aktion"=AK_SATK_Aktion."schreiben", "Cluster (in)"=cluster{"SATK":bool} {"SATK"=FALSE}) -> ()  [unwired: 9 in, 1 out]
      }
      frame "Pause" {
      }
      frame "Eco" {
        n241 = case shown="False" w357 {
          selector: w357 -> [_ w368]
          tunnel: [TRUE w368] -> w356
          frame False {
            n242 = local read "Status Analysatoren"() -> (w360:T2)
            n243 = Unbundle By Name(w360) -> ("FID"=w359:bool)
            n244 = case shown="True" w359 {
              frame False {
              }
              frame True {
                n245 = stacked-sequence {
                  frame #0 {
                    w362 = TRUE ("Standby")
                    n246 = Not(x=w362) -> (.not. x?=w363:bool)
                    n247 = call "STBY_MESSEN.vi"("Messen"=w363, "Aktion"=Aktion_STY_MES."setze MES") -> ()  [unwired: 10 in, 4 out]
                    n248 = call "STBY_MESSEN.vi"("Standby"=w362, "Aktion"=Aktion_STY_MES."setze STY") -> ()  [unwired: 10 in, 4 out]
                  }
                  frame #1 {
                    n249 = call "STBY_MESSEN.vi"("Case Nr."=2, "Aktion"=Aktion_STY_MES."MODBUS schreiben") -> ()  [unwired: 10 in, 4 out]
                  }
                }
              }
            }
          }
          frame True {
          }
        }
      }
      frame "Messen" {
        # "Freigabe"
        n250 = disable-structure shown="Deaktiviert" {
          frame Disabled {
            n251 = call "TOOLweb TRIGGER.vi"("action"=T36."startrun") -> ()  [unwired: 2 in, 5 out]
          }
          frame Enabled {
          }
        }
        n252 = Select(t=Zustaende."Messen vorbereiten" ("ausgewählte Funktion"), s=TRUE, f=w370) -> (s? t:f=w372:T16)
      }
      frame "Kalibrieren" {
        n253 = disable-structure shown="Deaktiviert" {
          frame Disabled {
            n254 = call "FGV System.vi"("Aktionen"=Aktioen_FGV_System."lesen") -> ("Optionen"=w379:T61)  [unwired: 12 in, 6 out]
            n255 = Unbundle By Name(w379) -> ("Reserve-Leakcheck vor Kal"=w378:bool)
            n256 = case shown="False" w378 {
              frame False {
                n257 = vi-ref "Auto Kalibrieren.lvlib:VI Auto Kalibrieren.vi"() -> (w381:refnum<vi>)
                n258 = call "VI Pop Up.vi"("VI Referenz"=w381) -> ()  [unwired: 10 in, 1 out]
              }
              frame True {
                n259 = vi-ref "Erweiterte Konfig.lvlib:Dichtheitstest.vi"() -> (w382:refnum<vi>)
                n260 = call "VI Pop Up.vi"("VI Referenz"=w382) -> ()  [unwired: 10 in, 1 out]
              }
            }
          }
          frame Enabled {
          }
        }
        n261 = disable-structure shown="Deaktiviert" {
          frame Disabled {
            n262 = vi-ref "Dichtheitstest.vi"() -> (w383:refnum<vi>)
            n263 = invoke class="VI" method="VI ausführen"(reference=w383, "Wait until done"=FALSE ("Warten bis beendet"), "Auto Dispose Ref"=TRUE ("Referenz automatisch schließen")) -> (reference out=w384:refnum<vi>)  [unwired: 2 in, 4 out]
            n264 = invoke class="VI" method="FP.Öffnen"(reference=w384) -> ()  [unwired: 4 in, 5 out]
          }
          frame Enabled {
          }
        }
        n265 = call "AK SATK FGV.vi"("Aktion"=AK_SATK_Aktion."initialisieren") -> ()  [unwired: 10 in, 1 out]
      }
      frame "Spülen Filter" {
      }
      frame "Spülen Leitung" {
      }
      frame "Umgebungsluft" {
      }
      frame "0-Gas" {
        n266 = case shown="False" w396 {
          selector: w396 -> [_ w411]
          tunnel: [TRUE w411] -> w395
          frame False {
            n267 = call "FGV FT-IR Parameter.vi"("Aktion"=FGV_FT-IR_Aktionen."lesen") -> ("Ausgangs-Cluster"=w403:T63)  [unwired: 11 in, 7 out]
            n268 = call "FGV System.vi"("Aktionen"=Aktioen_FGV_System."lesen") -> ("Optionen"=w407:T61)  [unwired: 12 in, 6 out]
            n269 = call "Kommunikation Stoerung.vi"("Aktionen"=Aktionen_Kommunikation_Stoerung."lesen") -> ("Störung Messgerät"=w406:T64)  [unwired: 10 in]
            n270 = Unbundle By Name(w403) -> ("Spektrum loggen aktiv?"=w401:bool)
            n271 = Unbundle By Name(w407) -> ("log 0-Gas"=w400:bool)
            n272 = Unbundle By Name(w406) -> ("FT-IR Komm"=w405:bool)
            n273 = Not(x=w405) -> (.not. x?=w399:bool)
            n274 = Compound Arithmetic op=AND(w401, w400, w399) -> (w402:bool)
            n275 = case shown="True" w402 {
              selector: w402 -> [_ w410]
              frame False {
              }
              frame True {
                n276 = call "TOOLweb SET LABFILE Enabled.vi"("Enabled"=w410) -> ()  [unwired: 2 in, 5 out]
              }
            }
          }
          frame True {
          }
        }
        n277 = call "FGV Trigger.vi"("Aktion"=Aktionen_Trigger."Trigger prüfen") -> ()  [unwired: 7 in, 4 out]
      }
      frame "Cal-Gas" {
        n278 = case shown="False" w415 {
          selector: w415 -> [_ w430]
          tunnel: [TRUE w430] -> w414
          frame False {
            n279 = call "FGV FT-IR Parameter.vi"("Aktion"=FGV_FT-IR_Aktionen."lesen") -> ("Ausgangs-Cluster"=w422:T63)  [unwired: 11 in, 7 out]
            n280 = call "FGV System.vi"("Aktionen"=Aktioen_FGV_System."lesen") -> ("Optionen"=w426:T61)  [unwired: 12 in, 6 out]
            n281 = call "Kommunikation Stoerung.vi"("Aktionen"=Aktionen_Kommunikation_Stoerung."lesen") -> ("Störung Messgerät"=w425:T64)  [unwired: 10 in]
            n282 = Unbundle By Name(w422) -> ("Spektrum loggen aktiv?"=w420:bool)
            n283 = Unbundle By Name(w426) -> ("log 0-Gas"=w419:bool)
            n284 = Unbundle By Name(w425) -> ("FT-IR Komm"=w424:bool)
            n285 = Not(x=w424) -> (.not. x?=w418:bool)
            n286 = Compound Arithmetic op=AND(w420, w419, w418) -> (w421:bool)
            n287 = case shown="True" w421 {
              selector: w421 -> [_ w429]
              frame False {
              }
              frame True {
                n288 = call "TOOLweb SET LABFILE Enabled.vi"("Enabled"=w429) -> ()  [unwired: 2 in, 5 out]
              }
            }
          }
          frame True {
          }
        }
        n289 = call "FGV Trigger.vi"("Aktion"=Aktionen_Trigger."Trigger prüfen") -> ()  [unwired: 7 in, 4 out]
      }
      frame "-------------" {
      }
      frame "Init 1" {
        n290 = call "Zykluszeiterfassung.vi"("Aktionen"=Zykluszeiterfassung_Aktionen."init") -> ()  [unwired: 10 in, 1 out]
        n291 = control-ref of="Permanent"() -> (w437:refnum<vi>)
        n292 = control-ref of="Mitte"() -> (w438:refnum<vi>)
        n293 = control-ref of="Fensterbereich"() -> (w434:refnum<vi>)
        n294 = call "Bildwechsel.vi"("Referenz Permanent"=w437, "Referenz Mitte"=w438, "nächstes Bild"=Bild-Auswahl."Initialisieren") -> ()  [unwired: 4 in, 5 out]
        n295 = call "Scrollbar einschalten.vi"("Aktion"=T38."Init", "Fensterbereich"=w434) -> ()  [unwired: 10 in]
      }
      frame "Init 2" {
        n296 = control-ref of="Funktionstasten"() -> (w442:refnum<vi>)
        n297 = stacked-sequence {
          tunnel: [_ w450 _ _ _] -> w443
          frame #0 {
            n298 = call "FGV Stoermeldungsdatei.vi"("Aktionen"=FGV_Stoerungsdatei_Aktionen."laden") -> ()  [unwired: 5 in, 6 out]
          }
          frame #1 {
            n299 = call "Betriebsdaten Laden-Speichern.vi"("Betriebsdaten"=Betriebsdaten_Aktionen."Laden") -> ("error IO"=w450:errorcluster, "Ausgangs-Cluster"=w451:T65)  [unwired: 1 in, 8 out]
            n300 = local write "Status Analysatoren"(w451) -> ()
          }
          frame #2 {
            n301 = call "FGV Gasliste.vi"("Aktionen"=FGV_FT-IR_Gasliste_Aktionen."lesen") -> ("Aktuelle Gasliste gesamt"=w453:T3[])  [unwired: 8 in, 2 out]
            n302 = call "AK Namen.vi"("Aktionen"=AK_Namen_Aktionen."lesen") -> ("AK Namen"=w455:string[])  [unwired: 7 in, 3 out]
            n303 = call "AK Namen.vi"("Aktionen"=AK_Namen_Aktionen."Liste erstellen", "AK Namen"=w455, "Aktuelle Gasliste FT-IR"=w453) -> ()  [unwired: 5 in, 4 out]
          }
          frame #3 {
            n304 = call "FGV System.vi"("Aktionen"=Aktioen_FGV_System."lesen") -> ("Optionen"=w459:T61)  [unwired: 12 in, 6 out]
            n305 = Unbundle By Name(w459) -> ("Verticale Scrollbar aktiv"=w458:bool)
            n306 = case shown="True" w458 {
              frame True {
                n307 = call "Scrollbar einschalten.vi"("Aktion"=T38."scroll V aktiv") -> ()  [unwired: 11 in]
              }
              frame False {
                n308 = call "Scrollbar einschalten.vi"("Aktion"=T38."scroll V inaktiv") -> ()  [unwired: 11 in]
              }
            }
          }
          frame #4 {
            n309 = call "Bildwechsel.vi"("nächstes Bild"=Bild-Auswahl."Grafik") -> ()  [unwired: 3 in, 8 out]
          }
        }
        n310 = call "FGV-Funktionstasten.vi"("Aktion"=Funktionstasten-Aktion."Manuell") -> ()  [unwired: 7 in, 8 out]
        n311 = call "FGV-Erweiterte Bedienung.vi"("Aktion"=FGV_Erweiterte_Bedienung_Aktion."Initialisieren") -> ()  [unwired: 9 in, 2 out]
        n312 = call "FGV-Funktionstasten.vi"("Referenz"=w442, "Zustand"=Zustaende."Standby", "Aktion"=Funktionstasten-Aktion."Initialisieren") -> ()  [unwired: 5 in, 8 out]
        n313 = disable-structure shown="SysLogAktiv==TRUE" {
          disable-tunnel: w443 -> [w465 _]
          frame condition #0 (active) {
            n314 = call "Syslog Interface PC.vi"("Fehler (in)"=w465, "Cluster (in)"=T19 {"FehlermeldungsCode"=3, "ErfolgsmeldungsCode"=3, "ParameterListenString"="", "Anzeige"=FALSE, "SysLogIcon"=enum."Warnung", "intern"=FALSE}) -> ()  [unwired: 9 in, 1 out]
          }
          frame condition #1 {
          }
        }
      }
      frame "Init 3" {
        # "#Option10xSpanAuto"
        n315 = vi-ref "VI Gaszuordnung.vi"() -> (w494:refnum<vi>)
        n316 = vi-ref "ARN Test Konfig v2.vi"() -> (w491:refnum<vi>)
        n317 = vi-ref "EPA 1065.lvlib:Dichtheitstest 1065-345.lvlib:Konfig Leak Check.vi"() -> (w490:refnum<vi>)
        n318 = vi-ref "EPA 1065.lvlib:Interference verificaton 1065-366.lvlib:VI Interference Konfig.vi"() -> (w489:refnum<vi>)
        n319 = vi-ref "EPA 1065.lvlib:T90 Test 1065-308.lvlib:T90 Test Konfig.vi"() -> (w488:refnum<vi>)
        n320 = vi-ref "EPA 1065.lvlib:Interference verificaton 1065-375.lvlib:VI Interference Konfig.vi"() -> (w483:refnum<vi>)
        n321 = vi-ref "EPA 1065.lvlib:Gas Analyzer Drift 1065-550.lvlib:Drift Verification Konfig.vi"() -> (w472:refnum<vi>)
        n322 = vi-ref "Linearisierung v2.lvlib:VI Linearisierung v2.vi"() -> (w470:refnum<vi>)
        n323 = vi-ref "EPA 1065.lvlib:HovaCAL Interference verificaton.lvlib:VI Interference Konfig.vi"() -> (w467:refnum<vi>)
        n324 = call "SubVI ausfuehren.vi"("Referenz"=w494) -> ("vi reference"=w497:refnum<vi>)  [unwired: 10 in]
        n325 = call "SubVI ausfuehren.vi"("Referenz"=w491) -> ("vi reference"=w487:refnum<vi>)  [unwired: 10 in]
        n326 = call "SubVI ausfuehren.vi"("Referenz"=w490) -> ("vi reference"=w486:refnum<vi>)  [unwired: 10 in]
        n327 = call "SubVI ausfuehren.vi"("Referenz"=w489) -> ("vi reference"=w485:refnum<vi>)  [unwired: 10 in]
        n328 = call "SubVI ausfuehren.vi"("Referenz"=w488) -> ("vi reference"=w484:refnum<vi>)  [unwired: 10 in]
        n329 = call "SubVI ausfuehren.vi"("Referenz"=w483) -> ("vi reference"=w482:refnum<vi>)  [unwired: 10 in]
        n330 = call "SubVI ausfuehren.vi"("Referenz"=w472) -> ("vi reference"=w471:refnum<vi>)  [unwired: 10 in]
        n331 = call "SubVI ausfuehren.vi"("Referenz"=w470) -> ("vi reference"=w469:refnum<vi>)  [unwired: 10 in]
        n332 = call "SubVI ausfuehren.vi"("Referenz"=w467) -> ("vi reference"=w466:refnum<vi>)  [unwired: 10 in]
        n333 = Build Array(w497, w487, w486, w485, w484, w482, w471, w469, w466) -> (w496:refnum<vi>[])
        n334 = call "FGV System.vi"("Aktionen"=Aktioen_FGV_System."lesen") -> ("Optionen"=w473:T61)  [unwired: 12 in, 6 out]
        n335 = disable-structure shown="LP_Anlage==TRUE, Standard" {
          disable-tunnel: [TRUE ("PNS?") w501] -> w480
          disable-tunnel: [T45 {"Analysator Auswahl"=0, "Analysator Auswahl 2"=0, "Analysator Auswahl 3"=0, "Analysator Auswahl 4"=0, "Analysator Auswahl 5"=0, "Analysator Auswahl 6"=0, "Analysator Auswahl 7"=0, "Analysator Auswahl 8"=0, "Analysator Auswahl 9"=0, "Analysator Auswahl 10"=0, "Analysator Auswahl 11"=0, "Analysator Auswahl 12"=0} ("Analysator Auswahl") w503] -> w474
          disable-tunnel: w473 -> [_ w502]
          frame condition #0 (active) {
          }
          frame condition #1 {
            n336 = Unbundle By Name(w502) -> ("PNS?"=w501:bool)
            n337 = call "FGV CalGas.vi"("Aktionen"=FGV_CalGas_Aktionen."lesen") -> ("Analysator Auswahl"=w503:T45)  [unwired: 6 in, 4 out]
          }
        }
        n338 = Current VI's Menubar() -> (w493:refnum<k9>)
        n339 = call "SubVIs abbrechen.vi"("Aktionen"=enum16{"Setzen", "abbrechen"}."Setzen", "vi referenzen"=w496) -> ()  [unwired: 10 in]
        n340 = call "Runtime Menue Text aendern.vi"("Menüreferenz"=w493) -> ("Fehler (Ausgang)"=w468:errorcluster)  [unwired: 10 in]
        n341 = Bundle By Name(cluster=w473, "PNS?"=w480) -> (w478:T61)
        n342 = call "FGV System.vi"("Optionen"=w478, "Aktionen"=Aktioen_FGV_System."Optionen schreiben") -> ("error out"=w477:errorcluster)  [unwired: 11 in, 6 out]
        n343 = call "FGV CalGas.vi"("Aktionen"=FGV_CalGas_Aktionen."Analysator Auswahl", "Analysator Auswahl"=w474) -> ()  [unwired: 5 in, 5 out]
        n344 = call "FGV System.vi"("error in (no error)"=w477, "Aktionen"=Aktioen_FGV_System."speichern") -> ()  [unwired: 11 in, 7 out]
      }
      frame "Init 4" {
        n345 = Current VI's Menubar() -> (w507:refnum<k9>)
        n346 = disable-structure shown="FID==FALSE&&PMA==FALSE, Standard" {
          disable-tunnel: [w528 w535] -> w513
          disable-tunnel: w507 -> [w528 w534]
          frame condition #0 {
            w533 = TRUE
            n347 = Not(x=w533) -> (.not. x?=w532:bool)
            n348 = property on="Status Analysatoren" class="Cluster (strikt)"("Visible"=w533) -> (error out=w531:errorcluster)  [unwired: 2 in, 1 out]
            n349 = property on="Aktuelles Rezept" class="Str (strikt)"("Visible"=w532) -> (error out=w529:errorcluster)  [unwired: 2 in, 1 out]
            n350 = Merge Errors(w531, w529) -> (w530:errorcluster)
            n351 = call <vilib>:"Clear Errors.vi"("error in (no error)"=w530) -> ()  [unwired: 5 in, 2 out]
          }
          frame condition #1 (active) {
            w542 = TRUE
            n352 = Not(x=w542) -> (.not. x?=w541:bool)
            n353 = property on="Aktuelles Rezept" class="Str (strikt)"("Visible"=w542) -> (error out=w538:errorcluster)  [unwired: 2 in, 1 out]
            n354 = property on="Status Analysatoren" class="Cluster (strikt)"("Visible"=w541) -> (error out=w539:errorcluster)  [unwired: 2 in, 1 out]
            n355 = Delete Menu Items(7:"Konfig CalGas" ("Menüpunkte"), 9:w534) -> (0:w537:errorcluster, 3:w535:refnum<k9>)  [unwired: 2 in]
            n356 = Merge Errors(w538, w539, w537) -> (w540:errorcluster)
            n357 = call <vilib>:"Clear Errors.vi"("error in (no error)"=w540) -> ()  [unwired: 5 in, 2 out]
          }
        }
        n358 = disable-structure shown="FID==FALSE" {
          disable-tunnel: w513 -> [w548 w550]
          disable-tunnel: [w548 w549] -> w512
          frame condition #0 {
          }
          frame condition #1 (active) {
            n359 = Delete Menu Items(7:"FID" ("Menüpunkte"), 9:w550) -> (0:w551:errorcluster, 3:w549:refnum<k9>)  [unwired: 2 in]
            n360 = call <vilib>:"Clear Errors.vi"("error in (no error)"=w551) -> ()  [unwired: 5 in, 2 out]
          }
        }
        n361 = call "TOOLweb TRIGGER.vi"("action"=Trigger_Aktionen."startrun") -> ()  [unwired: 2 in, 5 out]
        n362 = disable-structure shown="EPA_aktiv==FALSE" {
          disable-tunnel: w512 -> [w558 w560]
          disable-tunnel: [w558 w559] -> w511
          frame condition #0 {
          }
          frame condition #1 (active) {
            n363 = Delete Menu Items(7:"EPA §1065" ("Menüpunkte"), 9:w560) -> (0:w561:errorcluster, 3:w559:refnum<k9>)  [unwired: 2 in]
            n364 = call <vilib>:"Clear Errors.vi"("error in (no error)"=w561) -> ()  [unwired: 5 in, 2 out]
          }
        }
        n365 = disable-structure shown="PMA==FALSE" {
          disable-tunnel: w511 -> [w543 w545]
          disable-tunnel: [w543 w544] -> w510
          frame condition #0 {
          }
          frame condition #1 (active) {
            n366 = Delete Menu Items(7:"PMA" ("Menüpunkte"), 9:w545) -> (0:w546:errorcluster, 3:w544:refnum<k9>)  [unwired: 2 in]
            n367 = call <vilib>:"Clear Errors.vi"("error in (no error)"=w546) -> ()  [unwired: 5 in, 2 out]
          }
        }
        n368 = disable-structure shown="SysLogAktiv==FALSE" {
          disable-tunnel: w510 -> [w553 w555]
          disable-tunnel: [w553 w554] -> w506
          frame condition #0 (active) {
          }
          frame condition #1 {
            n369 = Delete Menu Items(7:"SysLog" ("Menüpunkte"), 9:w555) -> (0:w557:errorcluster, 3:w554:refnum<k9>)  [unwired: 2 in]
            n370 = call <vilib>:"Clear Errors.vi"("error in (no error)"=w557) -> ()  [unwired: 5 in, 2 out]
          }
        }
        n371 = disable-structure shown="CAN_Interface==TRUE, Standard" {
          disable-tunnel: w506 -> [_ w525]
          disable-tunnel: [_ w524] -> w505
          frame condition #0 {
          }
          frame condition #1 (active) {
            n372 = Delete Menu Items(7:"CAN Konfig" ("Menüpunkte"), 9:w525) -> (0:w527:errorcluster, 3:w524:refnum<k9>)  [unwired: 2 in]
            n373 = call <vilib>:"Clear Errors.vi"("error in (no error)"=w527) -> ()  [unwired: 5 in, 2 out]
          }
        }
        n374 = disable-structure shown="HovaCALInterferenceTest==FALSE, Standard" {
          disable-tunnel: w505 -> [_ w521]
          frame condition #0 {
          }
          frame condition #1 (active) {
            n375 = Delete Menu Items(7:"HovaCAL Querempfindlichkeitstest" ("Menüpunkte"), 9:w521) -> (0:w523:errorcluster)  [unwired: 2 in, 1 out]
            n376 = call <vilib>:"Clear Errors.vi"("error in (no error)"=w523) -> ()  [unwired: 5 in, 2 out]
          }
        }
        n377 = call "FGV Schedule Status.vi"("Aktion"=Aktion_FGV_Scheduler_Status."init") -> ()  [unwired: 13 in, 2 out]
        n378 = call "FGV CalGas.vi"("Aktionen"=FGV_CalGas_Aktionen."Def.CalGas", "Def.CalGas neu"=T48 {"Namen"={"Name"="Span 1", "Name 2"="Span 2", "Name 3"="Span 3", "Name 4"="", "Name 5"="", "Name 6"="", "Name 7"="", "Name 8"="", "Name 9"="", "Name 10"="", "Name 11"="", "Name 12"=""}, "Werte"={"Konzentration 1"=0.0, "Konzentration 2"=0.0, "Konzentration 3"=0.0, "Konzentration 4"=0.0, "Konzentration 5"=0.0, "Konzentration 6"=0.0, "Konzentration 7"=0.0, "Konzentration 8"=0.0, "Konzentration 9"=0.0, "Konzentration 10"=0.0, "Konzentration 11"=0.0, "Konzentration 12"=0.0}, "Werte 2"={"Konzentration 1"=0.0, "Konzentration 2"=0.0, "Konzentration 3"=0.0, "Konzentration 4"=0.0, "Konzentration 5"=0.0, "Konzentration 6"=0.0, "Konzentration 7"=0.0, "Konzentration 8"=0.0, "Konzentration 9"=0.0, "Konzentration 10"=0.0, "Konzentration 11"=0.0, "Konzentration 12"=0.0}, "Einheit"={"Einheit 1"=0, "Einheit 2"=0, "Einheit 3"=0, "Einheit 4"=0, "Einheit 5"=0, "Einheit 6"=0, "Einheit 7"=0, "Einheit 8"=0, "Einheit 9"=0, "Einheit 10"=0, "Einheit 11"=0, "Einheit 12"=0}, "Messbereiche"={"Messbereich 1"=0, "Messbereich 2"=0, "Messbereich 3"=0, "Messbereich 4"=0, "Messbereich 5"=0, "Messbereich 6"=0, "Messbereich 7"=0, "Messbereich 8"=0, "Messbereich 9"=0, "Messbereich 10"=0, "Messbereich 11"=0, "Messbereich 12"=0}}) -> ()  [unwired: 5 in, 5 out]
        n379 = call "Test Status.vi"("Aktion"=Aktion_Test_Status."init") -> ()  [unwired: 11 in, 4 out]
        n380 = call "FGV-Funktionstasten.vi"("Zustand"=Zustaende."Standby", "Aktion"=Funktionstasten-Aktion."Zustand setzen") -> ("ausgewählte Funktion"=w518:T16)  [unwired: 6 in, 7 out]
      }
      frame "Messen vorbereiten" {
        # "alles bereit ?"
        n381 = call "Kommunikation Stoerung.vi"("Aktionen"=Aktionen_Kommunikation_Stoerung."lesen") -> ("Störung Messgerät"=w565:T64)  [unwired: 10 in]
        n382 = Unbundle By Name(w565) -> ("FT-IR Komm"=w564:bool)
        n383 = case shown="True" w564 {
          frame False {
            n384 = call "FGV FT-IR Parameter.vi"("Aktion"=FGV_FT-IR_Aktionen."lesen") -> ("Ausgangs-Cluster"=w573:T63)  [unwired: 11 in, 7 out]
            n385 = Unbundle By Name(w573) -> ("Spektrum loggen aktiv?"=w572:bool)
            n386 = case shown="True" w572 {
              selector: w572 -> [_ w575]
              frame False {
              }
              frame True {
                n387 = call "TOOLweb SET LABFILE Enabled.vi"("Enabled"=w575) -> ()  [unwired: 2 in, 5 out]
              }
            }
          }
          frame True {
          }
        }
        n388 = call "FGV Trigger.vi"("Aktion"=Aktionen_Trigger."Trigger prüfen") -> ()  [unwired: 7 in, 4 out]
        n389 = Select(t=Zustaende."Messen durchführen", s=TRUE, f=w571) -> (s? t:f=w570:T16)
      }
      frame "Messen durchführen" {
      }
      frame "Exit" {
        w580 = TRUE
        n390 = stacked-sequence {
          frame #0 {
            n391 = call "Betriebsdaten Laden-Speichern.vi"("Betriebsdaten"=Betriebsdaten_Aktionen."Speichern") -> ("error IO"=w582:errorcluster)  [unwired: 1 in, 9 out]
            n392 = disable-structure shown="SysLogAktiv==TRUE" {
              disable-tunnel: w582 -> [w585 _]
              frame condition #0 (active) {
                n393 = call "Syslog Interface PC.vi"("Fehler (in)"=w585, "Cluster (in)"=T19 {"FehlermeldungsCode"=4, "ErfolgsmeldungsCode"=4, "ParameterListenString"="", "Anzeige"=FALSE, "SysLogIcon"=enum."Warnung", "intern"=FALSE}) -> ()  [unwired: 9 in, 1 out]
              }
              frame condition #1 {
              }
            }
          }
          frame #1 {
            n394 = call "SysLog PC store messages.vi"() -> ("Fehler (out)"=w586:errorcluster)  [unwired: 11 in]
            n395 = call <vilib>:"Clear Errors.vi"("error in (no error)"=w586) -> ()  [unwired: 5 in, 2 out]
          }
          frame #2 {
            n396 = call "Bildwechsel.vi"("nächstes Bild"=Bild-Auswahl."Beenden") -> ()  [unwired: 3 in, 8 out]
            n397 = call "FGV Stoermeldungen.vi"("Aktion"=FGV_Stoermeldungen_Aktion."Queue freigeben") -> ()  [unwired: 7 in, 4 out]
            n398 = call "SubVIs abbrechen.vi"("Aktionen"=enum16{"Setzen", "abbrechen"}."abbrechen") -> ()  [unwired: 11 in]
          }
        }
        n399 = shared-variable ".\\Variablen.lvlib\\Beenden"(w580) -> (error out=w578:errorcluster)  [unwired: 1 in]
      }
    }
    n400 = call "LN2 Extern Befuellung Warnung.vi"("Aktion"=Aktion_LN2_Extern_Befuellung_Warnung."blinken") -> ()  [unwired: 13 in, 2 out]
  }
  n401 = while {
    tunnel: [w617] -> w14
    tunnel: w4 -> [_]
    tunnel: w7 -> [w596]
    stop <- w618 stop-if-true
    n402 = call "FGV FT-IR Parameter.vi"("Aktion"=FGV_FT-IR_Aktionen."lesen") -> ("Current Recipe"=→"Aktuelles Rezept":string)  [unwired: 11 in, 7 out]
    n403 = Wait Until Next ms Multiple(millisecond multiple=u32 700 ("Vielfache von ms")) -> ()  [unwired: 1 out]
    n404 = call "FGV-Funktionstasten.vi"("Aktion"=Funktionstasten-Aktion."Lesen") -> ("Betriebsart"=w613:T58)  [unwired: 7 in, 7 out]
    n405 = disable-structure shown="LN2_Befuellung==FALSE" {
      disable-tunnel: [TRUE ("LN2 Befüllung") FALSE ("LN2 Befüllung")] -> w592
      frame condition #0 (active) {
      }
      frame condition #1 {
      }
    }
    n406 = case shown="\"Remote\"" w613 {
      tunnel: [T67."Enabled" ("Deaktiviert") T67."Disabled and Grayed Out" ("Deaktiviert") T67."Enabled" ("Deaktiviert")] -> w594
      frame "Manuell", Default {
      }
      frame "Remote" {
      }
      frame "Bitparallel" {
      }
    }
    n407 = disable-structure shown="cRio_aktiv==TRUE, Standard" {
      frame condition #0 (active) {
        n408 = call "FGV Lebt cRIO.vi"() -> ("lebt cRIO?"=w624:bool)  [unwired: 11 out]
        n409 = case shown="True" w624 {
          tunnel: [_ w625] -> w622
          frame False {
          }
          frame True {
            n410 = call "PC_Daten zu cRIO.vi"() -> ()  [unwired: 11 in]
            n411 = call "PC_Daten von cRIO.vi"() -> ("LifeBit"=w625:bool)  [unwired: 11 in]
          }
        }
        "LifeBit" <- w622
        n412 = call "Kommunikation Stoerung.vi"("Aktionen"=Aktionen_Kommunikation_Stoerung."Life Bit", "ERROR"=w622) -> ()  [unwired: 9 in, 1 out]
      }
      frame condition #1 {
      }
    }
    n413 = Select(t=T67."Enabled" ("Deaktiviert"), s=w592, f=T67."Disabled and Grayed Out" ("Deaktiviert")) -> (s? t:f=w600:T67)
    n414 = property on="Samplepoint" class="Ring (strikt)"("DisabledEnum"=w594) -> (error out=w603:errorcluster)  [unwired: 2 in, 1 out]
    n415 = property on="Aufschaltung Popup" class="Bool. (strikt)"("DisabledEnum"=w594) -> (error out=w593:errorcluster)  [unwired: 2 in, 1 out]
    n416 = property on="LN2-Behälter Spülen" class="Bool. (strikt)"("DisabledEnum"=w600) -> (error out=w604:errorcluster)  [unwired: 2 in, 1 out]
    n417 = Merge Errors(w604, w593, w603) -> (w602:errorcluster)
    n418 = call <vilib>:"Clear Errors.vi"("error in (no error)"=w602) -> ()  [unwired: 5 in, 2 out]
    n419 = call "FGV Passwortlevel.vi"("FGV Passwort Aktion"=FGV_Passwort_Aktion."lesen") -> ("aktueller Level"=w608:i16)  [unwired: 2 in, 8 out]
    "PW-Level" <- w608
    n420 = Equal To 0?(x=w608) -> (x = 0?=w606:bool)
    n421 = Select(t="LOGIN" ("Untertitel.Text"), s=w606, f="LOGOUT" ("Untertitel.Text")) -> (s? t:f=w598:string)
    n422 = call "Zeitstempel letzte Kalibrierungen.vi"("Aktionen"=Aktionen_Zeitstempel_speichern."lesen") -> ("Zeitstempeln"=w590:timestamp[])  [unwired: 10 in]
    n423 = Reverse 1D Array(array=w590) -> (reversed array=w611:timestamp[])
    n424 = call "Texte in VIs uebersetzen.vi"("Sprachliste"=w596, "String zum Übersetzen"=w598) -> ("String zum Übersetzen"=w597:string)  [unwired: 9 in, 4 out]
    n425 = shared-variable ".\\Variablen.lvlib\\Beenden"() -> (w618:bool, error out=w617:errorcluster)  [unwired: 1 out]
    n426 = Index Array(array=w611) -> (element=→"Letzte Kalibrierung":timestamp)  [unwired: 1 in]
    n427 = property on="login" class="Bool."("BoolText.Text"=w597) -> (error out=w610:errorcluster)  [unwired: 2 in, 1 out]
    n428 = call "FGV Status Analysatoren.vi"("Aktionen"=Aktion_Status_Analysatoren."Felder einfärben") -> ()  [unwired: 10 in, 1 out]
    n429 = call <vilib>:"Clear Errors.vi"("error in (no error)"=w610) -> ()  [unwired: 5 in, 2 out]
  }
  n430 = while {
    tunnel: [w636] -> w12
    tunnel: w4 -> [_]
    stop <- w637 stop-if-true
    n431 = Wait Until Next ms Multiple(millisecond multiple=u32 200 ("Vielfache von ms")) -> ()  [unwired: 1 out]
    n432 = call "FGV-Funktionstasten.vi"("Aktion"=Funktionstasten-Aktion."Lesen") -> ("ausgewählte Funktion"=w630:T16)  [unwired: 7 in, 7 out]
    n433 = Get Date/Time In Seconds() -> (seconds since 1Jan1904=w634:timestamp)
    n434 = To Double Precision Float(number=w630) -> (double precision float=w632:dbl)
    n435 = To Double Precision Float(number=w634) -> (double precision float=w633:dbl)
    n436 = Build Array(w632, w633) -> (w629:dbl[])
    n437 = disable-structure shown="cRio_aktiv==TRUE, Standard" {
      disable-tunnel: w629 -> [w639 _]
      frame condition #0 (active) {
        n438 = shared-variable "NI-cRIO9066-IAG\\Kommunikation mit PC.lvlib\\Zustand PC"(w639) -> (error out=w638:errorcluster)  [unwired: 1 out]
        n439 = call <vilib>:"Clear Errors.vi"("error in (no error)"=w638) -> ()  [unwired: 5 in, 2 out]
      }
      frame condition #1 {
      }
    }
    n440 = shared-variable ".\\Variablen.lvlib\\Beenden"() -> (w637:bool, error out=w636:errorcluster)  [unwired: 1 out]
  }
  n441 = flat-sequence {
    tunnel: w4 -> [_]
    tunnel: [w650] -> w13
    frame #0 {
      n442 = Wait (ms)(milliseconds to wait=u32 5000 ("Zu wartende ms")) -> ()  [unwired: 1 out]
    }
    frame #1 {
      n443 = disable-structure shown="Amium_PNS_aktiv==FALSE" {
        disable-tunnel: [w655 w656] -> w648
        frame condition #0 {
          n444 = call "VI AK Master Amium.vi"() -> ("error out"=w655:errorcluster)  [unwired: 11 in]
        }
        frame condition #1 (active) {
          n445 = call "VI Modbus KOMM .vi"() -> ("error out"=w656:errorcluster)  [unwired: 11 in]
        }
      }
      n446 = disable-structure shown="PMA==TRUE, Standard" {
        disable-tunnel: [w653 _] -> w643
        frame condition #0 {
          n447 = call "Komm Modbus PMA.vi"() -> ("error IO"=w653:errorcluster)  [unwired: 11 in]
        }
        frame condition #1 (active) {
        }
      }
      n448 = disable-structure shown="FID==TRUE, Standard" {
        disable-tunnel: [w654 _] -> w644
        frame condition #0 {
          n449 = call "Komm Modbus_F.vi"() -> ("error IO"=w654:errorcluster)  [unwired: 11 in]
        }
        frame condition #1 (active) {
        }
      }
      n450 = call "SchedulerVI.vi"() -> ("Fehler (Ausgang)"=w641:errorcluster)  [unwired: 11 in]
      n451 = call "HovaCal Komm.vi"() -> ("error IO"=w642:errorcluster)  [unwired: 11 in]
      n452 = call "VI AK.vi"() -> ("error out"=w649:errorcluster)  [unwired: 11 in]
      n453 = call "VI Stoermeldeverwaltung.vi"() -> ("error out"=w652:errorcluster)  [unwired: 11 in]
      n454 = call "VI Messdaten-Verteiler.vi"() -> ("error out"=w651:errorcluster)  [unwired: 11 in]
      n455 = call "In Datei Loggen.vi"() -> ("error out"=w647:errorcluster)  [unwired: 11 in]
      n456 = call "VI cRIO Ueberwachung.vi"() -> ("error out"=w646:errorcluster)  [unwired: 11 in]
      n457 = call "Gasteiler KommVI.vi"() -> ("error IO"=w645:errorcluster)  [unwired: 10 in, 1 out]
      n458 = Merge Errors(w652, w651, w649, w647, w648, w646, w645, w644, w643, w642, w641) -> (w650:errorcluster)
    }
  }
  n459 = call "Alle Frontpanels auslesen.vi"("Fehler (Eingang, kein Fehler)"=w1) -> ("Fehler (Ausgang)"=w3:errorcluster)  [unwired: 10 in]
  n460 = flat-sequence {
    tunnel: w4 -> [_]
    frame #0 {
      n461 = call "WebDav_main.vi"() -> ()  [unwired: 11 in, 1 out]
    }
  }
  n462 = while {
    tunnel: [w663] -> w6
    shift-right: [w658] -> _
    shift-left: w5 -> [w659]
    tunnel: w4 -> [_]
    tunnel: w3 -> [w657]
    tunnel: w2 -> [_]
    stop <- w664 stop-if-true
    n463 = Wait Until Next ms Multiple(millisecond multiple=u32 500 ("ms")) -> ()  [unwired: 1 out]
    n464 = call "FGV System Konstanten.vi"("Aktionen"=Aktioen_FGV_System_Konstanten."lesen", "error in"=w657) -> ("Sprachindex"=w658:u16)  [unwired: 5 in, 4 out]
    n465 = Not Equal?(x=w658, y=w659) -> (x != y?=w661:bool)
    n466 = shared-variable ".\\Variablen.lvlib\\Beenden"() -> (w664:bool, error out=w663:errorcluster)  [unwired: 1 out]
    n467 = case shown="True" w661 {
      tunnel: [_ w665] -> _
      frame False {
      }
      frame True {
        n468 = control-ref of="Funktionstasten"() -> (w666:refnum<vi>)
        n469 = Current VI's Menubar() -> (w667:refnum<k9>)
        n470 = call "Sprachumschaltung.vi"("menu reference"=w667, "Cluster (Eingang)"=w666) -> ("Fehler (Ausgang)"=w665:errorcluster)  [unwired: 9 in]
      }
    }
  }
  n471 = flat-sequence {
    tunnel: w14 -> [_]
    tunnel: w13 -> [_]
    tunnel: w12 -> [_]
    tunnel: w11 -> [_]
    tunnel: w8 -> [_]
    tunnel: w6 -> [_]
    frame #0 {
      n472 = shared-variable ".\\Variablen.lvlib\\Beenden"(FALSE ("Beenden")) -> (error out=w668:errorcluster)  [unwired: 1 out]
      n473 = Request Deallocation(TRUE ("Flag")) -> ()
      n474 = call <vilib>:"Clear Errors.vi"("error in (no error)"=w668) -> ()  [unwired: 5 in, 2 out]
    }
    frame #1 {
      n475 = call "Datei im Ordner des VI (EXE).vi"("Dateiname"="VI Leer.vi") -> ("EXE"=w671:bool)  [unwired: 8 in, 2 out]
      n476 = Quit LabVIEW(quit? (T)=w671) -> ()
    }
  }
